vi "Autonomous Independent.vi"() -> ()   [LabVIEW 2015]
doc: "This VI is called when autonomous begins, and will automatically be terminated when autonomous ends. You can carry out timed or sensor driven robot movement independently without needing to return to the caller."
uses:
  Goal Selection.ctl
  Defense Position.ctl
  Defenses.ctl
  Auto 2 Control.ctl
  <vilib>/Platform/TimedLoop/XDataNode/timing_clust.ctl
  <vilib>/Platform/TimedLoop/XDataNode/nitl_modes.ctl
  <vilib>/Platform/TimedLoop/XDataNode/wakeup.ctl
  <vilib>/Rock Robotics/WPI/MotorControl/WPI_MotorControlDeviceRef.ctl
  <vilib>/Rock Robotics/WPI/MotorControl/WPI_MotorControlType.ctl
  <vilib>/Rock Robotics/SystemInterfaces/DIO/FPGA_DIOPWMChannel.ctl
  <vilib>/Rock Robotics/WPI/PWM/WPI_PWMDeadband.ctl
  <vilib>/Rock Robotics/WPI/CAN/Jaguar/SubVIs/WPI_CANJaguar_ControlMode.ctl
  <vilib>/Rock Robotics/WPI/CAN/TalonSRX/WPI_CANTalonSRX_APIControlMode.ctl
  <userlib>/836-Library/Drive/Drive Code/Drive Code Support/Drive Code Bundle.ctl
  <userlib>/836-Library/Drive/Drive Code/Drive Code Support/Sensor Cluster.ctl
  <userlib>/836-Library/Drive/Drive Code/Drive Code Support/Camera Cluster.ctl
  <userlib>/836-Library/Drive/Drive Code/Drive Code Support/Drive Code Notifier.ctl
  <userlib>/836-Library/Drive/Drive Code/Drive Code Support/Drive Code Command.ctl
  <userlib>/836-Library/Drive/Drive Code/Logging Data.ctl
  <userlib>/836-Library/Pneumatics/Support Code/Pneumatics Notifier.ctl
  <userlib>/836-Library/Pneumatics/Support Code/Pneumatics Command.ctl
  <userlib>/836-Library/Pneumatics/Support Code/Pneumatics Status.ctl
  PortcullisStates.ctl
  <userlib>/836-Library/System/TDMSv2/TDMS Channel Info.ctl
  <userlib>/836-Library/System/TDMSv2/TDMS RT FIFO Packet.ctl
  <vilib>/Rock Robotics/Network Tables/NT Read Number.vi
  <vilib>/Rock Robotics/Network Tables/NT Read Boolean.vi
  <userlib>/836-Library/Drive/Drive Code/Drive Code Support/Drive Loop Do Nothing.vi
  <userlib>/836-Library/Pneumatics/Support Code/Pneumatics Command Set Periodic.vi
  <userlib>/836-Library/Drive/Drive Code/Drive Code Support/Drive Loop Drive Distance.vi
  <userlib>/836-Library/Drive/Drive Code/Drive Code Support/Drive Loop Drive Continuous.vi
  <userlib>/836-Library/Drive/Drive Code/Drive Code Support/Drive Loop Turn.vi
  <userlib>/836-Library/Drive/Drive Code/Drive Code Support/Drive Loop Hold Yaw.vi
  <userlib>/836-Library/Drive/Drive Code/Drive Code Support/Drive Loop Follow Camera.vi
  <userlib>/836-Library/Drive/Drive Code/Drive Code Support/Drive Loop Hold Position.vi
  <vilib>/platform/TimedLoop/XDataNode/XDataNode.xnode
  <vilib>/Platform/TimedLoop/XDataNode/XDNodeRunTimeDep.lvlib
panel:
  out "Y":dbl
  out "Desired X pos":dbl
  out "X pos":dbl
  out "XY Current":cluster{"X":dbl, "Y":dbl}={"X"=133.11, "Y"=0.0}
  out "Pitch":dbl(graph)=0.125
  out "Initial Pitch":dbl=1.25
  out "Stable Over Pitch":bool
  out "Over Pitch Th":bool
  out "Over Encoder Distance":bool
  out "Camera Valid":bool
  out "Robot Pitch":dbl
  out "Current Angle":dbl=-0.5625
  out "Desired Angle":dbl
  out "Initial Encoder Distance":dbl
  out "Current Distance":dbl=136.322655
  out "Target Distance":dbl
  out "Waveform Chart":dbl(graph)=19.0
  in  "Return Point":cluster{"X":dbl, "Y":dbl}
  in  "Tab Control":enum32{"Auto 2"}(tab)
  in  "Score Intake timer":dbl=3.0
  out "Defense to Cross":T1=enum."Portcullis"
  out "Starting Position":T2=enum."3"
  out "Goal Target":T3=enum."Stop"
  out "Starting IMU Yaw":dbl
  out "Current State":T4=enum."Stop"
  out "Pitch Up Detected":bool
  out "Pitch Down Detected":bool
  in  "Override Pitch Detection":bool
  in  "Backup Power":dbl=-1.0 format="%#_13g"
  in  "Tower Backup Offset":dbl=48.0 format="%#_13g"
  in  "Dist from Def":dbl=60.0
  in  "Portcullis Point":dbl=100.0
  in  "Portcullis Cross Power":dbl=0.6
  in  "Encoder Pause":dbl=0.4
  in  "Dist cross":dbl=120.0
  in  "Encoder not moving val":dbl=0.001
  in  "Eval Period for Port":dbl=0.8 format="%#_13g"
  # "00 - Start Delay\n01 - Defense Selection\n02 - Defense Crossing Detection\n03 - Drive Forward Past Defense\n04 - Turn to Rally Pt\n05 - Complete Rally pt Turn\n06 - Drive to Rally Pt\n07 - Finish Rally Pt Turn\n08 - Turn to Tower\n09 - Complete Turn to Tower\n10 - Drive to Twoer\n11 - Compelte Drive to Tower\n12 - Score\n13 - Back to Defense\n14 - Stop"
  # "Starting Values"
  # "Values from Dash"
  # "To Dash"
  # "TO QCP"
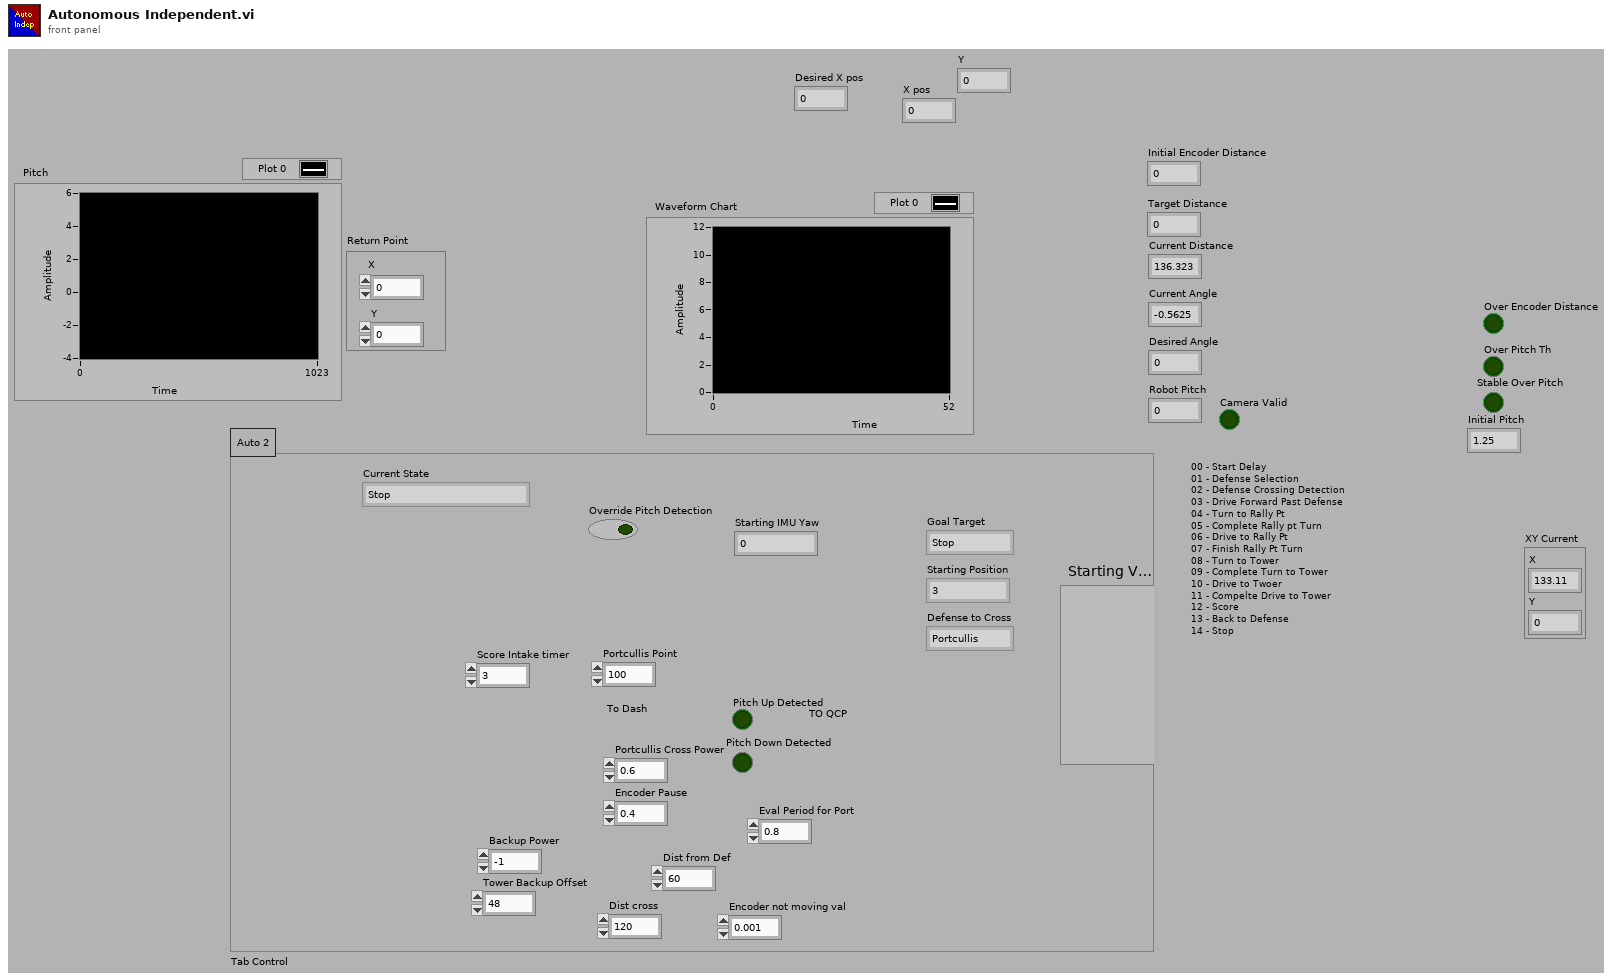
[diagram p1: front panel]
types:
  T1 = typedef "Defenses.ctl" = enum16{"Low Bar", "Rough Terrain", "Moat", "Rock Wall", "Cheval de Frise", "Portcullis", "Sally Port", "Drawbridge", "Ramparts"}
  T2 = typedef "Defense Position.ctl" = enum16{"1", "2", "3", "4", "5"}
  T3 = typedef "Goal Selection.ctl" = enum16{"Left Goal", "Right Goal", "Stop"}
  T4 = typedef "Auto 2 Control.ctl" = enum16{"Start Delay", "Defense Selection", "Defense Crossing Detection", "Drive Forward Past Defense", "Turn to Rally Pt", "Complete Rally Pt Turn", "Drive to Rally Pt", "Finish Drive to Rally Pt", "Turn to Tower", "Complete Turn to Tower", "Drive to Tower", "Complete Drive to Tower", "Score", "Parallel to Position", "Finish Backing Parallel to Pos", "Turn to Defense ", "Finish Turn to Def", "Back to Defense", "Finish Back to Defense", "Stop"}
  T5 = typedef "TDMS Channel Info.ctl" = cluster{"TDMS Data":T6, "TDMS RT FIFO":refnum<k33>}
  T6 = typedef "TDMS RT FIFO Packet.ctl" = cluster{"Group/CMD":i32, "Channel":i32, "Data":dbl}
  T7 = typedef "PortcullisStates.ctl" = enum16{"Drive up to Portcullis", "Intake Up", "Pause", "Cross", "Finish Cross"}
  T8 = typedef "WPI_MotorControlDeviceRef.ctl" = cluster{"DeviceStatus":errorcluster, "Type":T9, "PWM":cluster{"PWM Channel":T10, "DeadBand":T11}, "CAN":cluster{"Device Number":u8, "Control Mode":T12, "Semaphore":T13, "Max Vout":dbl, "TalonSRX Control Mode":T14}, "Invert":bool}
  T9 = typedef "WPI_MotorControlType.ctl" = enum16{"PWM", "CAN", "CANTalonSRX"}
  T10 = typedef "FPGA_DIOPWMChannel.ctl" = enum8{"PWM 0", "PWM 1", "PWM 2", "PWM 3", "PWM 4", "PWM 5", "PWM 6", "PWM 7", "PWM 8", "PWM 9", "PWM MXP 0", "PWM MXP 1", "PWM MXP 2", "PWM MXP 3", "PWM MXP 4", "PWM MXP 5", "PWM MXP 6", "PWM MXP 7", "PWM MXP 8", "PWM MXP 9", "Invalid"}
  T11 = typedef "WPI_PWMDeadband.ctl" = cluster{"Name":string, "maxPositivePwm":i32, "minPositivePwm":i32, "centerPwm":i32, "maxNegativePwm":i32, "minNegativePwm":i32, "angularRange":u16}
  T12 = typedef "WPI_CANJaguar_ControlMode.ctl" = enum8{"Percent VBus", "Current", "Speed", "Position", "Voltage"}
  T13 = typedef "Semaphore RefNum" = refnum<k1>
  T14 = typedef "WPI_CANTalonSRX_APIControlMode.ctl" = enum8{"Percent VBus", "Speed", "Position", "Slave", "Unchanged / Invalid", "Voltage Compensation", "Current", "Motion Profile"}
  T15 = typedef "Drive Code Bundle.ctl" = cluster{"Sensor Data":T16, "Drive Command rt fifo":refnum<k33>, "Logging Data":refnum<k33>}
  T16 = typedef "Sensor Cluster.ctl" = cluster{"Gyro Data":cluster{"Gyro RT FIFO":refnum<k33>, "Gyro Current":dbl, "Gyro Hold":dbl}, "Encoder Data":cluster{"Encoder RT FIFO":refnum<k33>, "Encoder Current":dbl, "Encoder Hold":dbl}, "Camera Data":cluster{"Camera RT FIFO":refnum<k33>, "Camera Current":T17}}
  T17 = typedef "Camera Cluster.ctl" = cluster{" Angle":dbl, "Valid":bool}
  T18 = typedef "Pneumatics Notifier.ctl" = cluster{"Command":refnum<notifier>, "Status":refnum<queue>}
  T19 = cluster{"intakeMotor":T8, "IMU Pitch":dbl, "Goal Target":T3, "IMU Yaw":dbl, "Initial Time":dbl, "Defense To Cross":T1, "Initial Position":T2, "Return Point":cluster{"X":dbl, "Y":dbl}, "Leave Tower?":bool, "Starting Delay":dbl, "IMU Roll":dbl, "Return Position":T2, "Drive Loop Cluster":T15, "Intake Command Cluster":T18}
  T20 = typedef "XDNodeRunTimeDep.lvlib/timing_clust.ctl" = cluster{"Expected End [f-1]":u64, "Actual End [f-1]":u64, "Finished Late? [f-1]":bool, "Expected End [i-1]":u64, "Actual End [i-1]":u64, "Finished Late? [i-1]":bool, "Expected Start [i]":u64, "Actual Start [i]":u64, "Expected Start [f]":u64, "Actual Start [f]":u64, "Source Name":string, "Structure Name":string, "Period":i64, "Deadline":i64, "Offset":i64, "Start":i64, "Priority":i32, "Timeout":i32, "Mode":T21, "Wakeup Reason":T22, "Error":errorcluster, "Source Type":string, "Secondary Source Type":string, "Global End Time":u64, "Global Start Time":u64, "Frame Duration":u64, "Iteration Duration":u64, "Assigned CPU":i32, "I/O Scan Engine Mode":u32}
  T21 = typedef "XDNodeRunTimeDep.lvlib/nitl_modes.ctl" = enum32{"No Change", "Process missed periods, maintain original phase", "Discard missed periods, maintain original phase", "Process missed periods, ignore original phase", "Discard missed periods, ignore original phase"}
  T22 = typedef "XDNodeRunTimeDep.lvlib/wakeup.ctl" = enum32{"Normal", "Aborted", "Asynchronous wakeup", "Timing source error", "Timed loop error", "Timeout"}
  T23 = typedef "Pneumatics Command.ctl" = enum16{"Nothing", "Forward", "Reverse", "Toggle"}
  T24 = cluster{"Rally Pt 2 X L":dbl, "Rally Pt 2 X L":dbl}
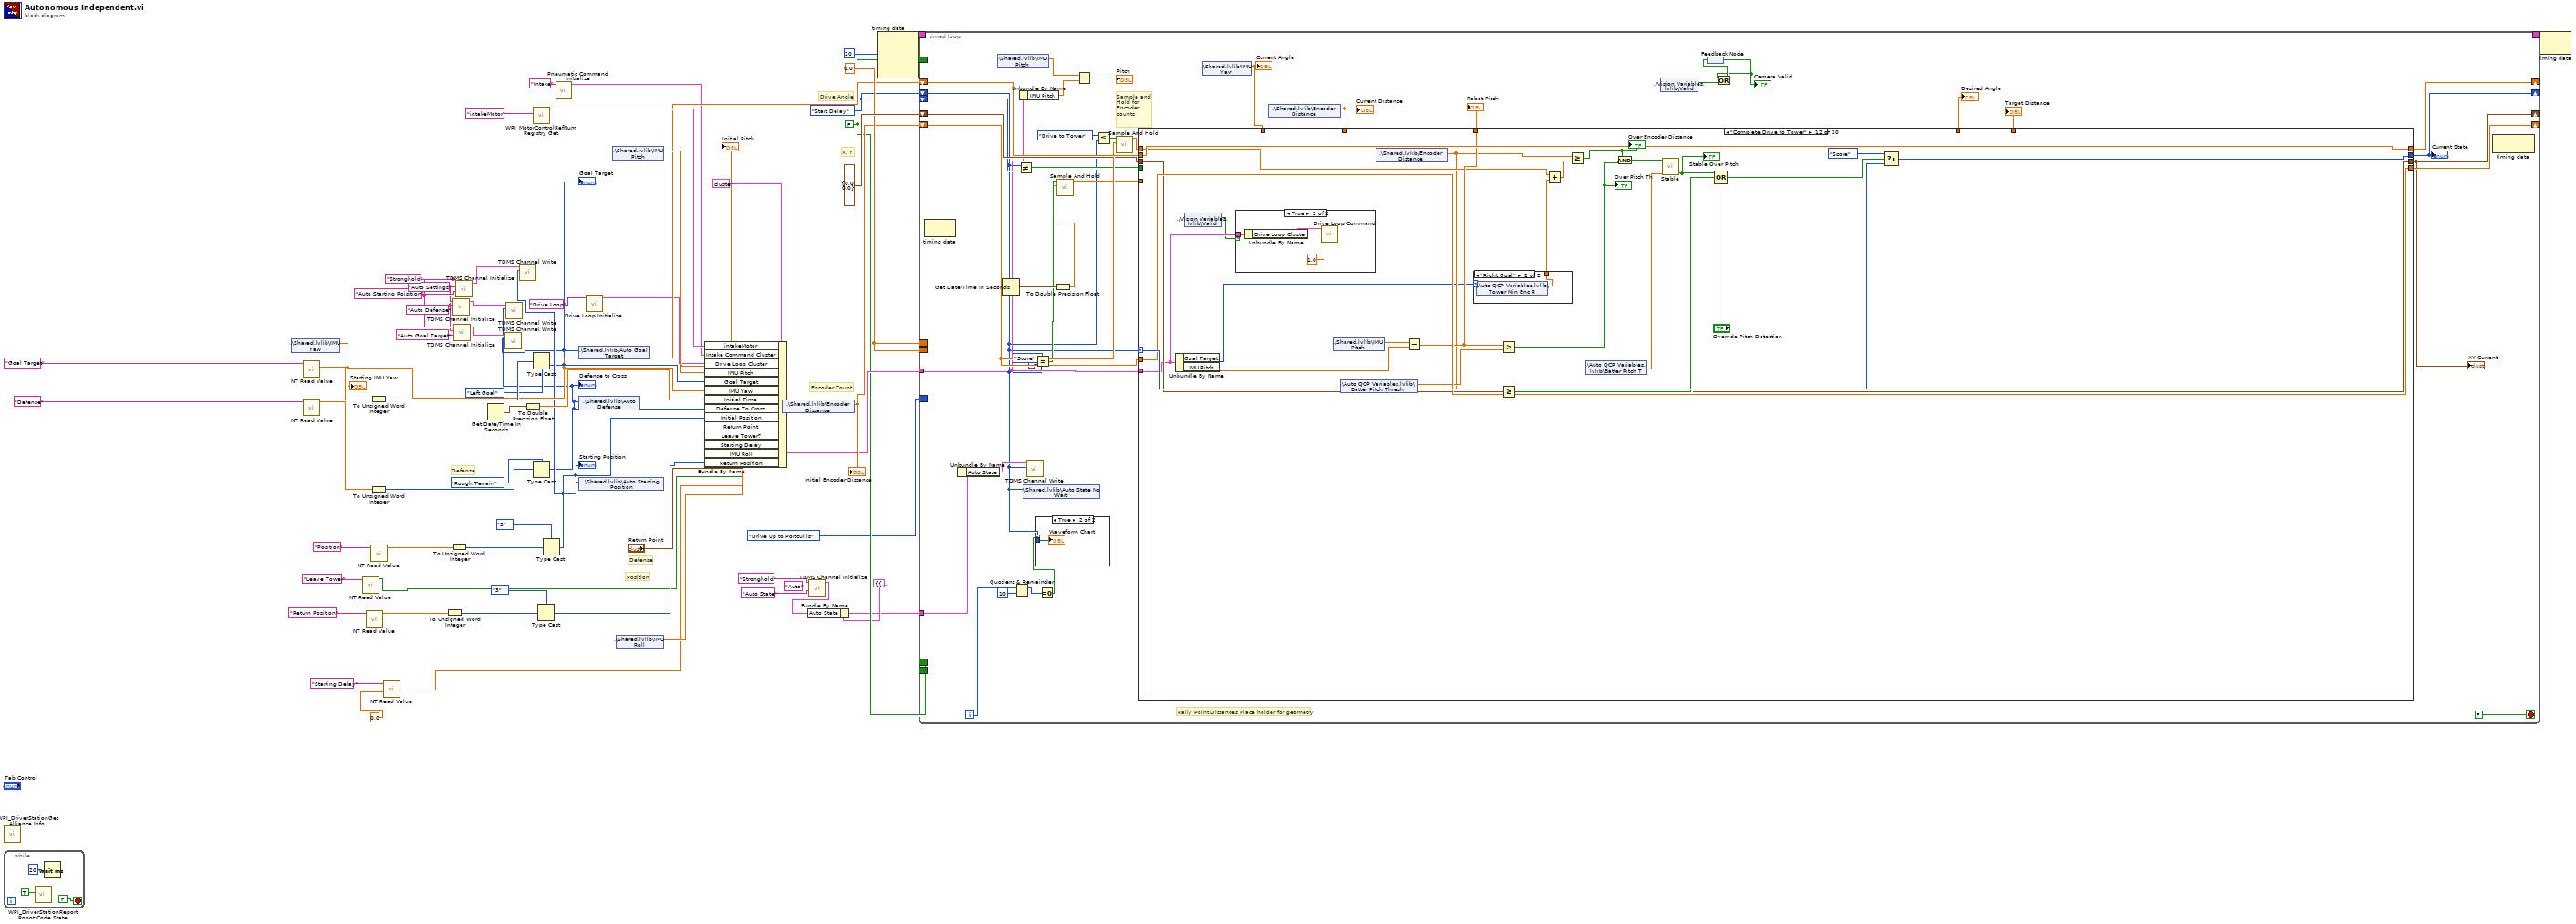
[diagram p0: block diagram]
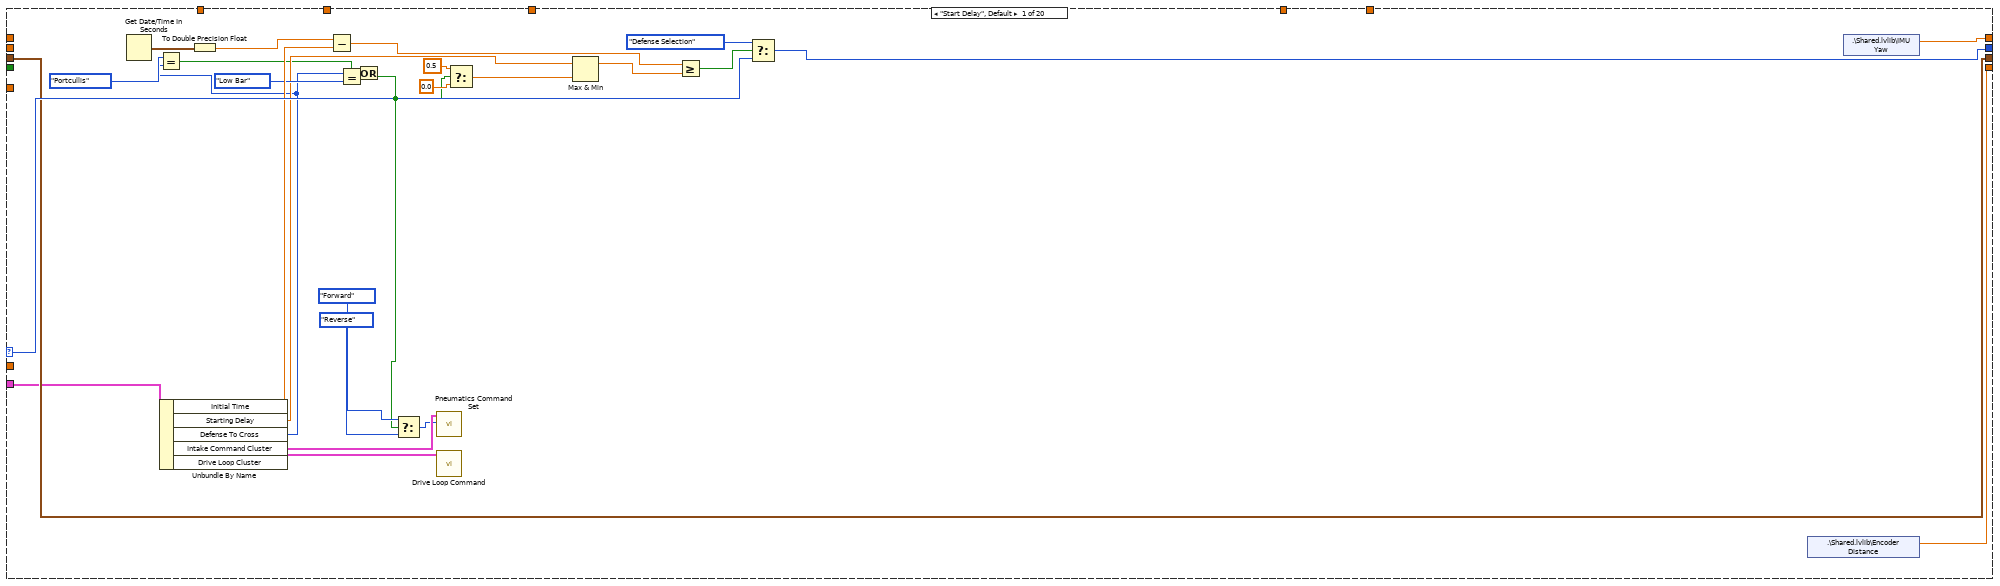
[diagram p3: hidden frame]
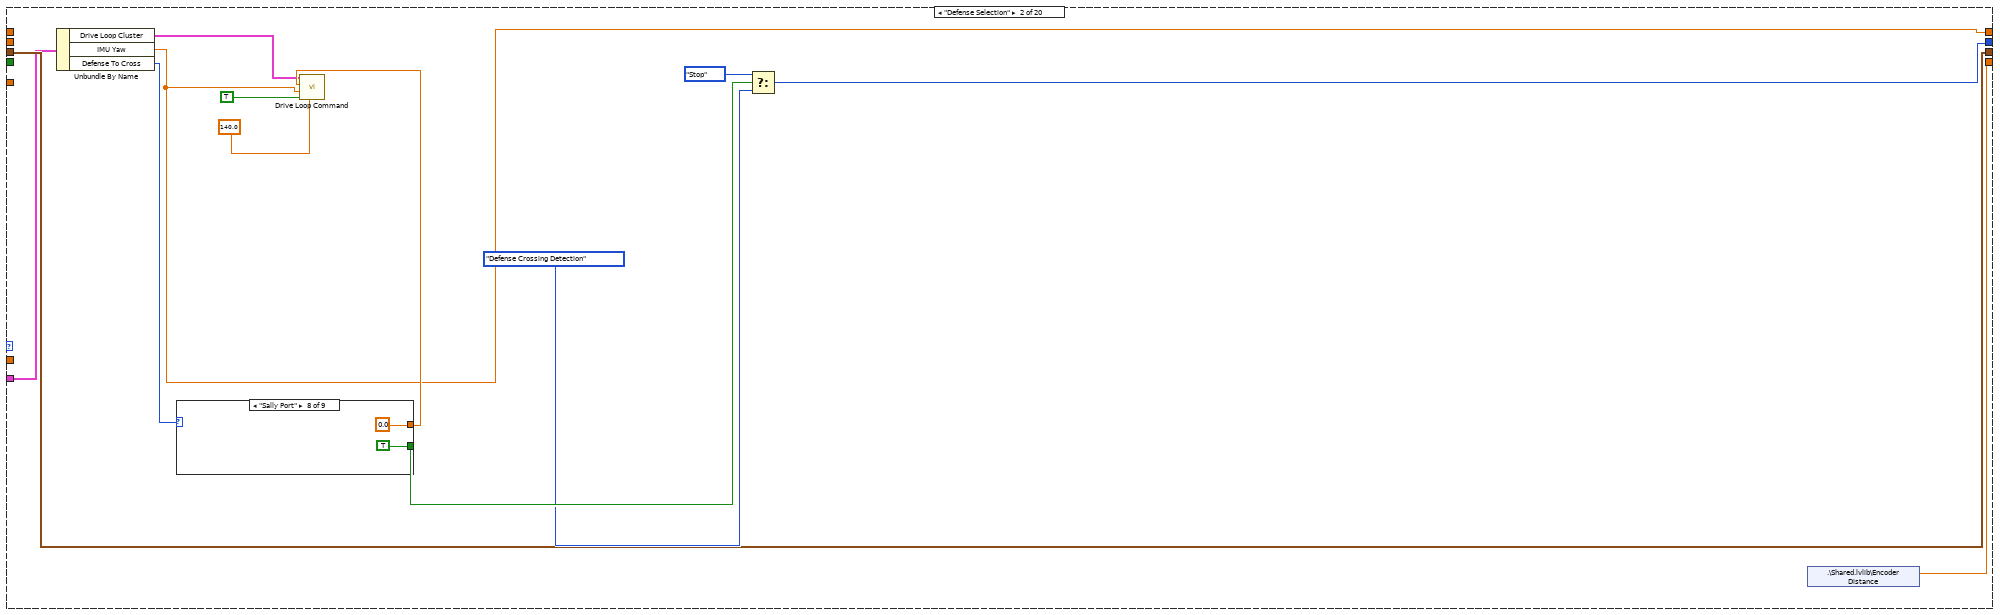
[diagram p4: hidden frame]
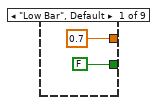
[diagram p5: hidden frame]
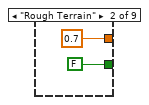
[diagram p6: hidden frame]
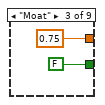
[diagram p7: hidden frame]
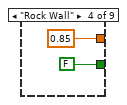
[diagram p8: hidden frame]
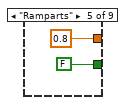
[diagram p9: hidden frame]
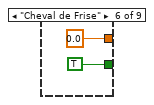
[diagram p10: hidden frame]
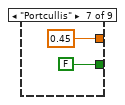
[diagram p11: hidden frame]
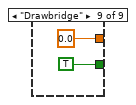
[diagram p12: hidden frame]
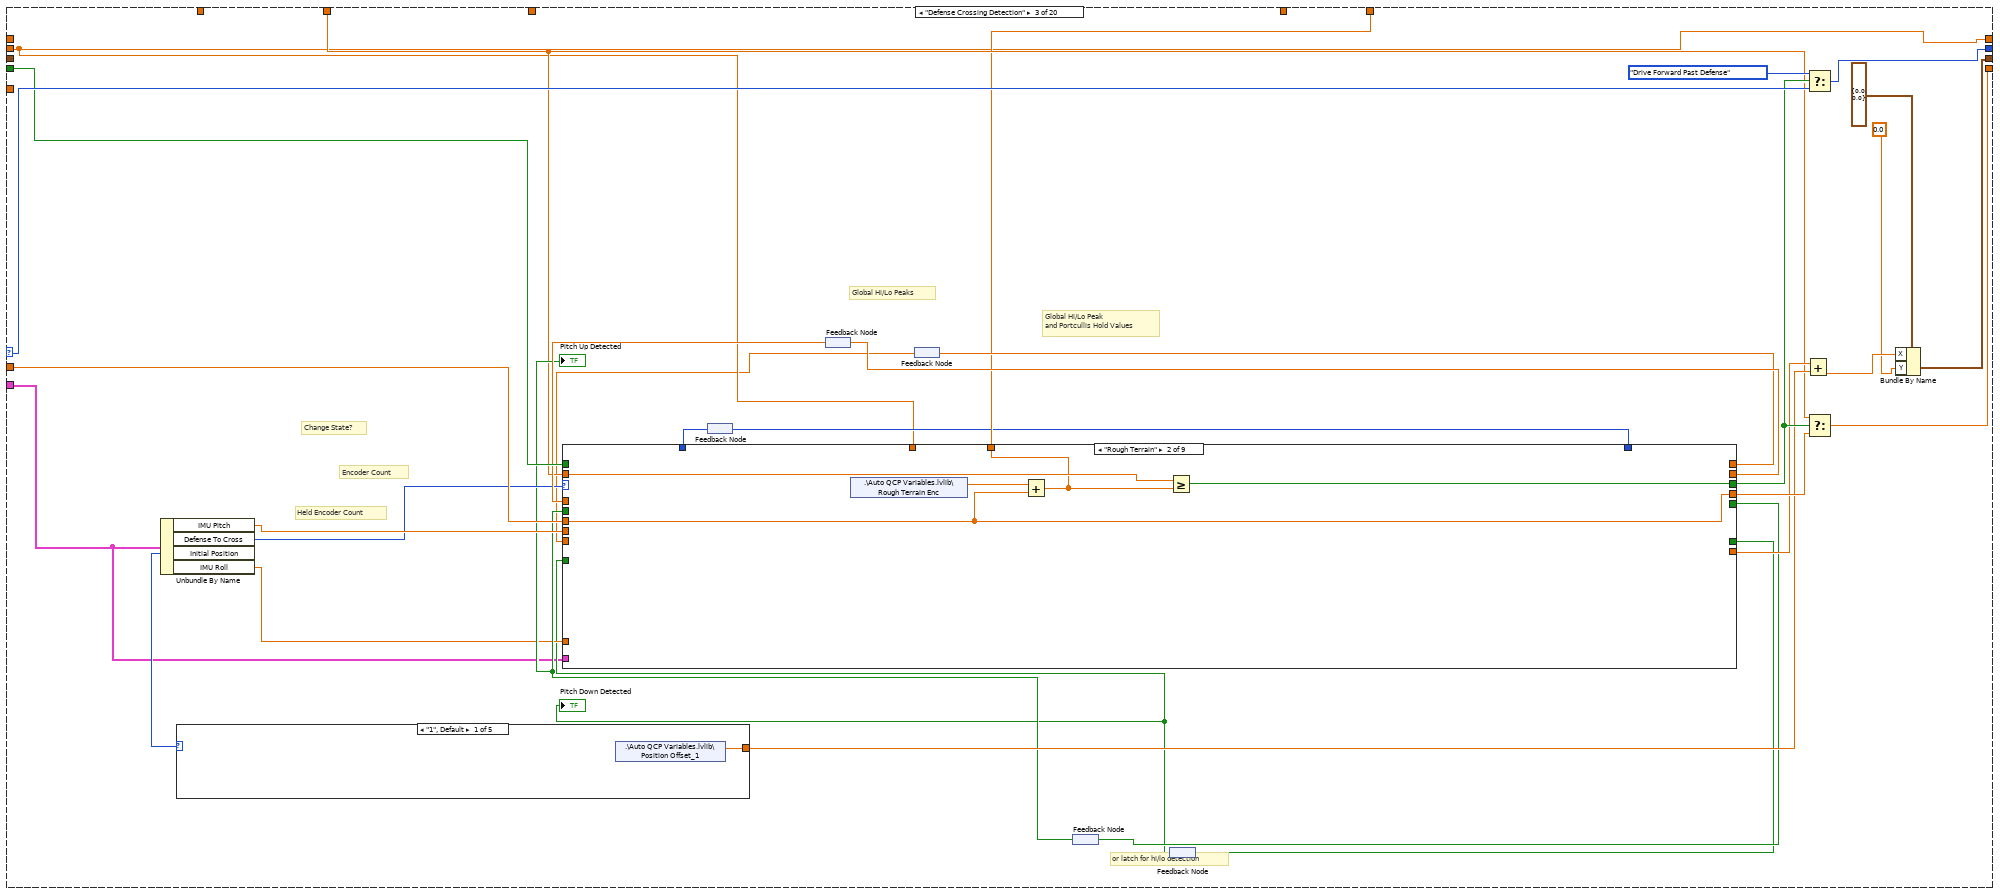
[diagram p13: hidden frame]
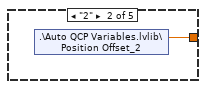
[diagram p14: hidden frame]
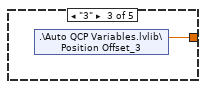
[diagram p15: hidden frame]
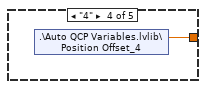
[diagram p16: hidden frame]
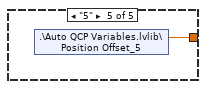
[diagram p17: hidden frame]
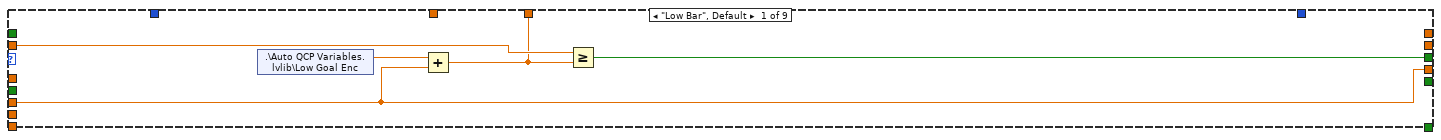
[diagram p18: hidden frame]
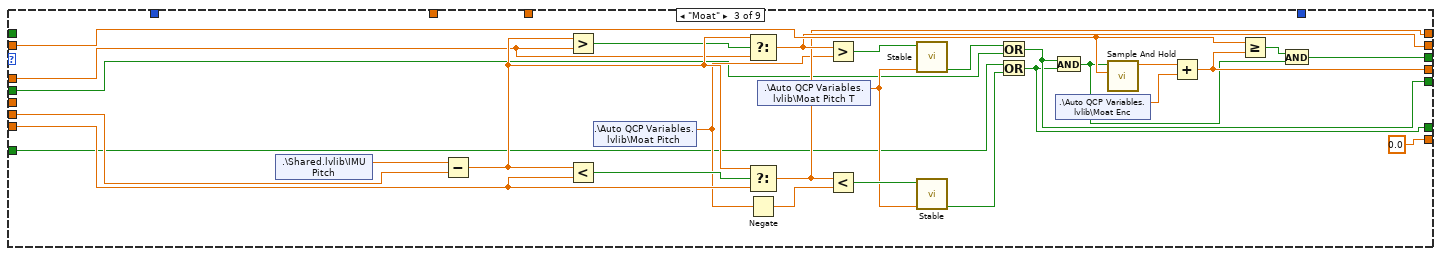
[diagram p19: hidden frame]
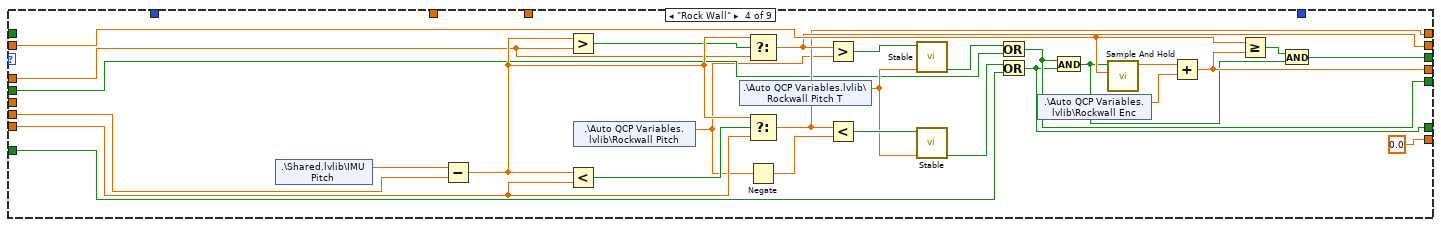
[diagram p20: hidden frame]
diagram:
  w9 = "Auto Settings" ("Group")
  w10 = "Stronghold" ("TDMS Name")
  w33 = FALSE
  w44 = 0.0 ("Double")
  w43 = Auto_2_Control."Start Delay"
  # "X, Y"
  # "Drive Angle"
  # "Encoder Count"
  # "Position"
  # "Defense"
  # "Defense"
  n1 = call <vilib>:"WPI_DriverStationGet Alliance Info.vi"() -> ()  [unwired: 12 out]
  n2 = while {
    stop <- FALSE stop-if-true
    n3 = call <vilib>:"WPI_DriverStationReport Robot Code State.vi"("Autonomous"=TRUE) -> ()  [unwired: 10 in, 1 out]
    n4 = Wait (ms)(milliseconds to wait=u32 20) -> ()  [unwired: 1 out]
  }
  n5 = shared-variable ".\\Shared.lvlib\\IMU Yaw"() -> (w37:dbl)  [unwired: 1 in, 1 out]
  "Starting IMU Yaw" <- w37
  n6 = call-poly <vilib>:"NT Read Value.vi"("Name"="Goal Target") -> ("Numeric"=w54:dbl)  [unwired: 9 in, 1 out]
  n7 = call-poly <vilib>:"NT Read Value.vi"("Name"="Defense") -> ("Numeric"=w60:dbl)  [unwired: 9 in, 1 out]
  n8 = call-poly <vilib>:"NT Read Value.vi"("Name"="Leave Tower") -> ("Boolean"=w27:bool)  [unwired: 9 in, 1 out]
  n9 = call-poly <vilib>:"NT Read Value.vi"("Name"="Return Position") -> ("Numeric"=w29:dbl)  [unwired: 9 in, 1 out]
  n10 = To Unsigned Word Integer(number=w54) -> (unsigned 16bit integer=w55:u16)
  n11 = To Unsigned Word Integer(number=w60) -> (unsigned 16bit integer=w59:u16)
  n12 = call-poly <vilib>:"NT Read Value.vi"("Name"="Position") -> ("Numeric"=w52:dbl)  [unwired: 9 in, 1 out]
  n13 = call-poly <vilib>:"NT Read Value.vi"("Default Value"=0.0, "Name"="Starting Delay") -> ("Numeric"=w23:dbl)  [unwired: 8 in, 1 out]
  n14 = To Unsigned Word Integer(number=w29) -> (unsigned 16bit integer=w31:u16)
  n15 = To Unsigned Word Integer(number=w52) -> (unsigned 16bit integer=w50:u16)
  n16 = call <userlib>:"TDMS Channel Initialize.vi"("Channel"="Auto Defense", "Group"=w9, "TDMS"=w10) -> ("TDMS Channel Info"=w5:T5)  [unwired: 8 in]
  n17 = call <userlib>:"TDMS Channel Initialize.vi"("Channel"="Auto Goal Target", "Group"=w9, "TDMS"=w10) -> ("TDMS Channel Info"=w4:T5)  [unwired: 8 in]
  n18 = call <userlib>:"TDMS Channel Initialize.vi"("Channel"="Auto Starting Poisition", "Group"=w9, "TDMS"=w10) -> ("TDMS Channel Info"=w6:T5)  [unwired: 8 in]
  n19 = Get Date/Time In Seconds() -> (seconds since 1Jan1904=w48:timestamp)
  n20 = To Double Precision Float(number=w48) -> (double precision float=w36:dbl)
  n21 = call <vilib>:"WPI_MotorControlRefNum Registry Get.vi"("refnum name"="intakeMotor") -> ("MotorControlDevRef"=w40:T8)  [unwired: 9 in, 1 out]
  n22 = Type Cast(type=Goal_Selection."Left Goal" ("Goal Target"), x=w55) -> (*(type *) &x=w1:T3)
  "Goal Target" <- w1
  n23 = call <userlib>:"TDMS Channel Write.vi"("Data"=w1, "TDMS Channel Info in"=w4) -> ()  [unwired: 9 in, 1 out]
  n24 = Type Cast(type=Defenses."Rough Terrain", x=w59) -> (*(type *) &x=w2:T1)
  "Defense to Cross" <- w2
  n25 = call <userlib>:"TDMS Channel Write.vi"("Data"=w2, "TDMS Channel Info in"=w5) -> ()  [unwired: 9 in, 1 out]
  n26 = Type Cast(type=Defense_Position."3", x=w31) -> (*(type *) &x=w28:T2)
  n27 = Type Cast(type=Defense_Position."3", x=w50) -> (*(type *) &x=w3:T2)
  "Starting Position" <- w3
  n28 = call <userlib>:"TDMS Channel Write.vi"("Data"=w3, "TDMS Channel Info in"=w6) -> ()  [unwired: 9 in, 1 out]
  n29 = call <userlib>:"Pneumatic Command Initialize.vi"("name (unnamed)"="Intake") -> ("Pneumatic Command Cluster"=w18:T18)  [unwired: 9 in, 1 out]
  n30 = shared-variable ".\\Shared.lvlib\\Auto Goal Target"(w1) -> ()  [unwired: 1 in, 1 out]
  n31 = shared-variable ".\\Shared.lvlib\\Auto Defense"(w2) -> ()  [unwired: 1 in, 1 out]
  n32 = shared-variable ".\\Shared.lvlib\\Auto Starting Position"(w3) -> ()  [unwired: 1 in, 1 out]
  n33 = call <userlib>:"Drive Loop Initialize.vi"("name (unnamed)"="Drive Loop") -> ("Drive Loop Cluster"=w21:T15)  [unwired: 9 in, 1 out]
  n34 = shared-variable ".\\Shared.lvlib\\IMU Pitch"() -> (w38:dbl)  [unwired: 1 in, 1 out]
  "Initial Pitch" <- w38
  n35 = shared-variable ".\\Shared.lvlib\\IMU Roll"() -> (w34:dbl)  [unwired: 1 in, 1 out]
  n36 = Bundle By Name(cluster=T19 {"intakeMotor"={"DeviceStatus"={"status"=FALSE, "code"=0, "source"=""}, "Type"=enum."PWM", "PWM"={"PWM Channel"=enum."Invalid", "DeadBand"={"Name"="", "maxPositivePwm"=0, "minPositivePwm"=0, "centerPwm"=0, "maxNegativePwm"=0, "minNegativePwm"=0, "angularRange"=0}}, "CAN"={"Device Number"=0, "Control Mode"=enum."Percent VBus", "Semaphore"=refnum, "Max Vout"=12.0, "TalonSRX Control Mode"=enum."Percent VBus"}, "Invert"=FALSE}, "IMU Pitch"=0.0, "Goal Target"=enum."Left Goal", "IMU Yaw"=0.0, "Initial Time"=0.0, "Defense To Cross"=enum."Low Bar", "Initial Position"=enum."3", "Return Point"={"X"=0.0, "Y"=0.0}, "Leave Tower?"=FALSE, "Starting Delay"=0.0, "IMU Roll"=0.0, "Return Position"=enum."3", "Drive Loop Cluster"={"Sensor Data"={"Gyro Data"={"Gyro RT FIFO"=refnum, "Gyro Current"=0.0, "Gyro Hold"=0.0}, "Encoder Data"={"Encoder RT FIFO"=refnum, "Encoder Current"=0.0, "Encoder Hold"=0.0}, "Camera Data"={"Camera RT FIFO"=refnum, "Camera Current"={" Angle"=0.0, "Valid"=FALSE}}}, "Drive Command rt fifo"=refnum, "Logging Data"=refnum}, "Intake Command Cluster"={"Command"=refnum, "Status"=refnum}}, "intakeMotor"=w40, "Intake Command Cluster"=w18, "Drive Loop Cluster"=w21, "IMU Pitch"=w38, "Goal Target"=w1, "IMU Yaw"=w37, "Initial Time"=w36, "Defense To Cross"=w2, "Initial Position"=w3, "Return Point"="Return Point", "Leave Tower?"=w27, "Starting Delay"=w23, "IMU Roll"=w34, "Return Position"=w28) -> (w39:T19)
  n37 = shared-variable ".\\Shared.lvlib\\Encoder Distance"() -> (w42:dbl)  [unwired: 1 in, 1 out]
  "Initial Encoder Distance" <- w42
  n38 = call <userlib>:"TDMS Channel Initialize.vi"("Channel"="Auto State", "Group"="Auto", "TDMS"="Stronghold" ("TDMS Name")) -> ("TDMS Channel Info"=w15:T5)  [unwired: 8 in]
  n39 = Bundle By Name(cluster=cluster{"Auto State":T5} {"Auto State"={"TDMS Data"={"Group/CMD"=0, "Channel"=0, "Data"=0.0}, "TDMS RT FIFO"=refnum}}, "Auto State"=w15) -> (w14:cluster{"Auto State":T5})
  n40 = node-c288(i64 20 ("Period")) -> (w47:T20)  [unwired: 3 in]
  n41 = timed-loop {
    timing: w47 -> [_]
    timing-out: [_] -> w46
    shift-right: [w92] -> _
    shift-left: w43 -> [w66]
    shift-right: [w102] -> _
    shift-left: w42 -> [w99]
    shift-right: [w100] -> _
    shift-left: w37 -> [w101]
    shift-right: [w95] -> _
    shift-left: cluster{"X":dbl, "Y":dbl} {"X"=0.0, "Y"=0.0} ("input cluster") -> [w96]
    shift-left: w43 -> [w94]
    border: w44 -> [_]
    border: w44 -> [_]
    tunnel: w39 -> [w78]
    border: w33 -> [_]
    border: w33 -> [_]
    border: w33 -> [_]
    border: PortcullisStates."Drive up to Portcullis" -> [_]
    tunnel: w14 -> [w68]
    i -> [w86]
    stop <- FALSE stop-if-true
    # "Sample and Hold for Encoder counts"
    # "Rally Point Distances Place holder for geometry"
    n42 = node-c288() -> ()  [unwired: 1 in, 1 out]
    n43 = Unbundle By Name(w68) -> ("Auto State"=w67:T5)
    n44 = shared-variable ".\\Shared.lvlib\\IMU Pitch"() -> (w77:dbl)  [unwired: 1 in, 1 out]
    n45 = Get Date/Time In Seconds() -> (seconds since 1Jan1904=w72:timestamp)
    n46 = Quotient & Remainder(x=w86, y=10) -> (x-y*floor(x/y)=w84:i32)  [unwired: 1 out]
    n47 = Not Equal?(x=w66, y=w94) -> (x != y?=w73:bool)
    n48 = Unbundle By Name(w78) -> ("IMU Pitch"=w76:dbl)
    n49 = shared-variable ".\\Shared.lvlib\\Auto State No Wait"(w66) -> ()  [unwired: 1 in, 1 out]
    n50 = call <userlib>:"TDMS Channel Write.vi"("Data"=w66, "TDMS Channel Info in"=w67) -> ()  [unwired: 9 in, 1 out]
    n51 = Equal?(x=w66, y=Auto_2_Control."Score") -> (x = y?=w69:bool)
    n52 = Equal To 0?(x=w84) -> (x = 0?=w83:bool)
    n53 = case shown="True" w83 {
      tunnel: w66 -> [_ w103]
      frame False {
      }
      frame True {
        "Waveform Chart" <- w103
      }
    }
    n54 = To Double Precision Float(number=w72) -> (double precision float=w71:dbl)
    n55 = call "Sample And Hold.vi"("Signal"=w71, "Condition"=w69) -> ("Signal Out"=w70:dbl)  [unwired: 9 in]
    n56 = Subtract(x=w77, y=w76) -> (x-y=→"Pitch":dbl)
    n57 = Less Or Equal?(x=Auto_2_Control."Drive to Tower", y=w66) -> (x <= y?=w93:bool)
    n58 = call "Sample And Hold.vi"("Signal"=w99, "Condition"=w93) -> ("Signal Out"=w98:dbl)  [unwired: 9 in]
    n59 = shared-variable ".\\Shared.lvlib\\IMU Yaw"() -> (w74:dbl)  [unwired: 1 in, 1 out]
    "Current Angle" <- w74
    n60 = shared-variable ".\\Shared.lvlib\\Encoder Distance"() -> (w89:dbl)  [unwired: 1 in, 1 out]
    "Current Distance" <- w89
    n61 = case shown="\"Complete Drive to Tower\"" w66 {
      selector: w66 -> [w127 _ w194 w377 _ w479 _ w502 _ w535 _ w574 w600 _ w627 _ w670 _ w703 _]
      tunnel: [w126 w141 w193 w376 w434 w482 Auto_2_Control."Finish Drive to Rally Pt" ("t") w504 Auto_2_Control."Complete Turn to Tower" ("t") w534 Auto_2_Control."Complete Drive to Tower" ("t") w573 w599 Auto_2_Control."Finish Backing Parallel to Pos" w634 Auto_2_Control."Finish Turn to Def" w672 Auto_2_Control."Finish Back to Defense" ("t") w701 Auto_2_Control."Stop"] -> w92
      tunnel: [w123 w140 w188 w372 w433 w478 w491 w498 w521 w533 w548 w566 w591 w613 w630 w658 w668 w690 w699 w711] -> w102
      tunnel: w99 -> [_ _ w191 w372 _ _ w495 w498 _ _ _ w566 _ w613 w630 _ _ w692 w699 w711]
      tunnel: [w122 w132 w165 w362 w418 w474 w488 w500 w508 w536 w547 w564 w592 w608 w622 w656 w669 w688 w700 w712] -> w100
      tunnel: w101 -> [_ _ w165 _ _ w474 w488 w500 _ w536 w547 w564 _ w608 w622 _ w669 w688 w700 w712]
      tunnel: w98 -> [_ _ _ _ _ _ _ _ _ _ _ w557 _ _ _ _ _ _ _ _]
      tunnel: w96 -> [w124 w139 _ w363 w432 w477 w494 w497 w510 w530 w546 w560 w590 w612 w632 w667 w683 w693 w704 w713]
      tunnel: [w124 w139 w186 w370 w421 w477 w494 w497 w509 w530 w546 w560 w590 w612 w631 w667 w683 w694 w704 w713] -> w95
      tunnel: w73 -> [_ _ w181 _ _ _ _ _ _ _ _ _ w581 _ _ _ _ _ _ w707]
      tunnel: w78 -> [w121 w138 w163 w367 w431 _ w492 _ w519 _ w544 w552 w586 w614 w640 w666 w681 w695 _ w709]
      tunnel: w89 -> [_ _ w169 _ _ _ _ _ _ _ _ _ _ _ w644 w658 _ _ w698 _]
      tunnel: [_ _ w168 w364 _ _ w491 _ _ _ _ _ _ _ _ _ _ _ w699 _] -> w88
      tunnel: [_ _ _ w362 w418 w474 _ _ _ _ _ _ _ _ _ _ _ _ _ _] -> w87
      tunnel: [_ _ _ _ _ _ _ _ _ _ _ w559 _ _ _ _ _ _ _ _] -> w82
      tunnel: w74 -> [_ _ _ _ _ _ _ _ _ _ _ _ _ _ _ _ w682 _ _ _]
      tunnel: w70 -> [_ _ _ _ _ _ _ _ _ _ _ _ w582 _ _ _ _ _ _ _]
      frame "Start Delay", Default {
        n62 = Get Date/Time In Seconds() -> (seconds since 1Jan1904=w131:timestamp)
        n63 = Unbundle By Name(w121) -> ("Initial Time"=w120:dbl, "Starting Delay"=w115:dbl, "Defense To Cross"=w111:T1, "Intake Command Cluster"=w108:T18, "Drive Loop Cluster"=w109:T15)
        n64 = Equal?(x=Defenses."Portcullis" ("y"), y=w111) -> (x = y?=w110:bool)
        n65 = To Double Precision Float(number=w131) -> (double precision float=w130:dbl)
        n66 = Subtract(x=w130, y=w120) -> (x-y=w129:dbl)
        n67 = Equal?(x=w111, y=Defenses."Low Bar") -> (x = y?=w113:bool)
        n68 = Or(x=w110, y=w113) -> (x .or. y?=w104:bool)
        n69 = Select(t=Pneumatics_Command."Forward" ("Solenoid Command"), s=w104, f=Pneumatics_Command."Reverse" ("Solenoid Command")) -> (s? t:f=w107:T23)
        n70 = call-poly <userlib>:"Pneumatics Command Set.vi"("Solenoid Command"=w107, "Cluster"=w108) -> ()  [unwired: 9 in, 1 out]
        n71 = call-poly <userlib>:"Drive Loop Command.vi"("Drive Loop Cluster"=w109) -> ()  [unwired: 11 in]
        n72 = Select(t=0.5, s=w104, f=0.0) -> (s? t:f=w116:dbl)
        n73 = Max & Min(x=w115, y=w116) -> (max(x,y)=w114:dbl)  [unwired: 1 out]
        n74 = Greater Or Equal?(x=w129, y=w114) -> (x >= y?=w128:bool)
        n75 = Select(t=Auto_2_Control."Defense Selection", s=w128, f=w127) -> (s? t:f=w126:T4)
        n76 = shared-variable ".\\Shared.lvlib\\Encoder Distance"() -> (w123:dbl)  [unwired: 1 in, 1 out]
        n77 = shared-variable ".\\Shared.lvlib\\IMU Yaw"() -> (w122:dbl)  [unwired: 1 in, 1 out]
      }
      frame "Defense Selection" {
        n78 = Unbundle By Name(w138) -> ("Drive Loop Cluster"=w134:T15, "IMU Yaw"=w132:dbl, "Defense To Cross"=w137:T1)
        n79 = case shown="\"Sally Port\"" w137 {
          tunnel: [0.7 ("Power") 0.7 ("Power") 0.75 ("Power") 0.85 ("Power") 0.8 ("Power") 0.0 ("Power") 0.45 ("Power") 0.0 ("Power") 0.0 ("Power")] -> w135
          tunnel: [FALSE FALSE FALSE FALSE FALSE TRUE FALSE TRUE TRUE] -> w144
          frame "Low Bar", Default {
          }
          frame "Rough Terrain" {
          }
          frame "Moat" {
          }
          frame "Rock Wall" {
          }
          frame "Ramparts" {
          }
          frame "Cheval de Frise" {
          }
          frame "Portcullis" {
          }
          frame "Sally Port" {
          }
          frame "Drawbridge" {
          }
        }
        n80 = call-poly <userlib>:"Drive Loop Command.vi"("Distance"=140.0, "Absolute Angle? 4"=TRUE, "Angle 3"=w132, "Power 3"=w135, "Drive Loop Cluster"=w134) -> ()  [unwired: 7 in]
        n81 = Select(t=Auto_2_Control."Stop", s=w144, f=Auto_2_Control."Defense Crossing Detection") -> (s? t:f=w141:T4)
        n82 = shared-variable ".\\Shared.lvlib\\Encoder Distance"() -> (w140:dbl)  [unwired: 1 in, 1 out]
      }
      frame "Defense Crossing Detection" {
        # "or latch for hi/lo detection"
        # "Global Hi/Lo Peak\nand Portcullis Hold Values"
        # "Global Hi/Lo Peaks"
        # "Change State?"
        # "Encoder Count"
        # "Held Encoder Count"
        n83 = Unbundle By Name(w163) -> ("IMU Pitch"=w177:dbl, "Defense To Cross"=w176:T1, "Initial Position"=w175:T2, "IMU Roll"=w171:dbl)
        n84 = case shown="\"1\", Default" w175 {
          tunnel: [w195 w196 w197 w198 w199] -> w185
          frame "1", Default {
            n85 = shared-variable ".\\Auto QCP Variables.lvlib\\Position Offset_1"() -> (w195:dbl)  [unwired: 1 in, 1 out]
          }
          frame "2" {
            n86 = shared-variable ".\\Auto QCP Variables.lvlib\\Position Offset_2"() -> (w196:dbl)  [unwired: 1 in, 1 out]
          }
          frame "3" {
            n87 = shared-variable ".\\Auto QCP Variables.lvlib\\Position Offset_3"() -> (w197:dbl)  [unwired: 1 in, 1 out]
          }
          frame "4" {
            n88 = shared-variable ".\\Auto QCP Variables.lvlib\\Position Offset_4"() -> (w198:dbl)  [unwired: 1 in, 1 out]
          }
          frame "5" {
            n89 = shared-variable ".\\Auto QCP Variables.lvlib\\Position Offset_5"() -> (w199:dbl)  [unwired: 1 in, 1 out]
          }
        }
        n90 = feedback #1() -> (w167:T7)
        n91 = feedback #2() -> (w179:dbl)
        n92 = feedback #3() -> (w164:dbl)
        n93 = feedback #4() -> (w173:bool)
        "Pitch Up Detected" <- w173
        n94 = feedback #5() -> (w170:bool)
        "Pitch Down Detected" <- w170
        n95 = case shown="\"Rough Terrain\"" w176 {
          tunnel: w169 -> [w204 w208 w233 w262 w266 _ w307 _ _]
          tunnel: w191 -> [w202 w209 _ _ _ _ w303 _ _]
          tunnel: [w203 w207 w214 w241 w275 _ w305 _ FALSE] -> w189
          tunnel: [w202 w209 w231 w260 w292 _ w303 _ _] -> w190
          tunnel: [_ _ 0.0 0.0 w282 w298 0.0 ("Double") _ _] -> w184
          tunnel: w177 -> [_ _ w221 w251 w283 _ _ _ _]
          tunnel: w181 -> [_ _ _ _ _ _ _ _ _]
          tunnel: [_ _ w225 w254 w286 _ _ _ _] -> w180
          tunnel: w179 -> [_ _ w229 w258 w291 _ _ _ _]
          tunnel: [_ _ w224 w253 w287 _ w302 _ _] -> w178
          tunnel: w164 -> [_ _ w228 w257 w290 _ w306 _ _]
          tunnel: [_ _ w215 w245 w279 _ _ _ _] -> w174
          tunnel: w173 -> [_ _ w216 w246 w278 _ _ _ _]
          tunnel: [_ _ w212 w239 w277 _ _ _ _] -> w172
          tunnel: w170 -> [_ _ w211 w238 w276 _ _ _ _]
          tunnel: w171 -> [_ _ _ _ w272 _ _ _ _]
          tunnel: [w200 w205 _ _ _ _ _ _ _] -> w168
          tunnel: w167 -> [_ _ _ _ _ _ w310 _ _]
          tunnel: [_ _ _ _ _ _ w309 _ _] -> w166
          tunnel: w165 -> [_ _ _ _ _ _ w308 _ _]
          tunnel: w163 -> [_ _ _ _ _ _ w301 _ _]
          frame "Low Bar", Default {
            n96 = shared-variable ".\\Auto QCP Variables.lvlib\\Low Goal Enc"() -> (w201:dbl)  [unwired: 1 in, 1 out]
            n97 = Add(x=w201, y=w202) -> (x+y=w200:dbl)
            n98 = Greater Or Equal?(x=w204, y=w200) -> (x >= y?=w203:bool)
          }
          frame "Rough Terrain" {
            n99 = shared-variable ".\\Auto QCP Variables.lvlib\\Rough Terrain Enc"() -> (w206:dbl)  [unwired: 1 in, 1 out]
            n100 = Add(x=w206, y=w209) -> (x+y=w205:dbl)
            n101 = Greater Or Equal?(x=w208, y=w205) -> (x >= y?=w207:bool)
          }
          frame "Moat" {
            n102 = shared-variable ".\\Shared.lvlib\\IMU Pitch"() -> (w236:dbl)  [unwired: 1 in, 1 out]
            n103 = Subtract(x=w236, y=w221) -> (x-y=w237:dbl)
            n104 = Greater?(x=w237, y=w229) -> (0:w227:bool)
            n105 = Less?(x=w237, y=w228) -> (x < y?=w226:bool)
            n106 = shared-variable ".\\Auto QCP Variables.lvlib\\Moat Pitch"() -> (w223:dbl)  [unwired: 1 in, 1 out]
            n107 = Select(t=w237, s=w227, f=w229) -> (s? t:f=w225:dbl)
            n108 = Select(t=w237, s=w226, f=w228) -> (s? t:f=w224:dbl)
            n109 = Negate(x=w223) -> (-x=w222:dbl)
            n110 = shared-variable ".\\Auto QCP Variables.lvlib\\Moat Pitch T"() -> (w218:dbl)  [unwired: 1 in, 1 out]
            n111 = Greater?(x=w225, y=w223) -> (0:w220:bool)
            n112 = Less?(x=w224, y=w222) -> (x < y?=w219:bool)
            n113 = call <userlib>:"Stable.vi"("Eval Period (sec)"=w218, "Signal Input"=w220) -> ("Stable"=w217:bool)  [unwired: 9 in]
            n114 = call <userlib>:"Stable.vi"("Eval Period (sec)"=w218, "Signal Input"=w219) -> ("Stable"=w210:bool)  [unwired: 9 in]
            n115 = Or(x=w217, y=w216) -> (x .or. y?=w215:bool)
            n116 = Or(x=w211, y=w210) -> (x .or. y?=w212:bool)
            n117 = And(x=w215, y=w212) -> (x .and. y?=w213:bool)
            n118 = shared-variable ".\\Auto QCP Variables.lvlib\\Moat Enc"() -> (w235:dbl)  [unwired: 1 in, 1 out]
            n119 = call "Sample And Hold.vi"("Signal"=w233, "Condition"=w213) -> ("Signal Out"=w234:dbl)  [unwired: 9 in]
            n120 = Add(x=w234, y=w235) -> (x+y=w231:dbl)
            n121 = Greater Or Equal?(x=w233, y=w231) -> (x >= y?=w232:bool)
            n122 = And(x=w232, y=w213) -> (x .and. y?=w214:bool)
          }
          frame "Rock Wall" {
            n123 = shared-variable ".\\Shared.lvlib\\IMU Pitch"() -> (w264:dbl)  [unwired: 1 in, 1 out]
            n124 = Subtract(x=w264, y=w251) -> (x-y=w265:dbl)
            n125 = Greater?(x=w265, y=w258) -> (0:w256:bool)
            n126 = Less?(x=w265, y=w257) -> (x < y?=w255:bool)
            n127 = shared-variable ".\\Auto QCP Variables.lvlib\\Rockwall Pitch"() -> (w244:dbl)  [unwired: 1 in, 1 out]
            n128 = shared-variable ".\\Auto QCP Variables.lvlib\\Rockwall Pitch T"() -> (w248:dbl)  [unwired: 1 in, 1 out]
            n129 = Select(t=w265, s=w256, f=w258) -> (s? t:f=w254:dbl)
            n130 = Select(t=w265, s=w255, f=w257) -> (s? t:f=w253:dbl)
            n131 = Negate(x=w244) -> (-x=w252:dbl)
            n132 = Greater?(x=w254, y=w244) -> (0:w250:bool)
            n133 = Less?(x=w253, y=w252) -> (x < y?=w249:bool)
            n134 = call <userlib>:"Stable.vi"("Eval Period (sec)"=w248, "Signal Input"=w250) -> ("Stable"=w247:bool)  [unwired: 9 in]
            n135 = call <userlib>:"Stable.vi"("Eval Period (sec)"=w248, "Signal Input"=w249) -> ("Stable"=w242:bool)  [unwired: 9 in]
            n136 = Or(x=w247, y=w246) -> (x .or. y?=w245:bool)
            n137 = Or(x=w242, y=w238) -> (x .or. y?=w239:bool)
            n138 = shared-variable ".\\Auto QCP Variables.lvlib\\Rockwall Enc"() -> (w243:dbl)  [unwired: 1 in, 1 out]
            n139 = And(x=w245, y=w239) -> (x .and. y?=w240:bool)
            n140 = call "Sample And Hold.vi"("Signal"=w262, "Condition"=w240) -> ("Signal Out"=w263:dbl)  [unwired: 9 in]
            n141 = Add(x=w263, y=w243) -> (x+y=w260:dbl)
            n142 = Greater Or Equal?(x=w262, y=w260) -> (x >= y?=w261:bool)
            n143 = And(x=w261, y=w240) -> (x .and. y?=w241:bool)
          }
          frame "Ramparts" {
            n144 = shared-variable ".\\Shared.lvlib\\IMU Pitch"() -> (w297:dbl)  [unwired: 1 in, 1 out]
            n145 = shared-variable ".\\Shared.lvlib\\IMU Roll"() -> (w273:dbl)  [unwired: 1 in, 1 out]
            n146 = Subtract(x=w297, y=w283) -> (x-y=w270:dbl)
            n147 = Subtract(x=w273, y=w272) -> (x-y=w271:dbl)
            n148 = Subtract(x=w270, y=w271) -> (x-y=w269:dbl)
            n149 = shared-variable ".\\Auto QCP Variables.lvlib\\Ramparts Pitch"() -> (w284:dbl)  [unwired: 1 in, 1 out]
            n150 = Less?(x=w269, y=w290) -> (x < y?=w288:bool)
            n151 = Greater?(x=w269, y=w291) -> (0:w289:bool)
            n152 = shared-variable ".\\Auto QCP Variables.lvlib\\Ramparts Pitch T"() -> (w267:dbl)  [unwired: 1 in, 1 out]
            n153 = Select(t=w269, s=w288, f=w290) -> (s? t:f=w287:dbl)
            n154 = Select(t=w269, s=w289, f=w291) -> (s? t:f=w286:dbl)
            n155 = Negate(x=w284) -> (-x=w285:dbl)
            n156 = Less?(x=w287, y=w285) -> (x < y?=w281:bool)
            n157 = Greater?(x=w286, y=w284) -> (0:w296:bool)
            n158 = call <userlib>:"Stable.vi"("Eval Period (sec)"=w267, "Signal Input"=w281) -> ("Stable"=w280:bool)  [unwired: 9 in]
            n159 = call <userlib>:"Stable.vi"("Eval Period (sec)"=w267, "Signal Input"=w296) -> ("Stable"=w268:bool)  [unwired: 9 in]
            n160 = Or(x=w278, y=w280) -> (x .or. y?=w279:bool)
            n161 = Or(x=w268, y=w276) -> (x .or. y?=w277:bool)
            n162 = shared-variable ".\\Auto QCP Variables.lvlib\\Ramparts Enc"() -> (w295:dbl)  [unwired: 1 in, 1 out]
            n163 = And(x=w279, y=w277) -> (x .and. y?=w274:bool)
            n164 = call "Sample And Hold.vi"("Signal"=w266, "Condition"=w274) -> ("Signal Out"=w294:dbl)  [unwired: 9 in]
            n165 = shared-variable ".\\Auto QCP Variables.lvlib\\Ramparts Offset"() -> (w282:dbl)  [unwired: 1 in, 1 out]
            n166 = Add(x=w294, y=w295) -> (x+y=w292:dbl)
            n167 = Greater Or Equal?(x=w266, y=w292) -> (x >= y?=w293:bool)
            n168 = And(x=w274, y=w293) -> (x .and. y?=w275:bool)
          }
          frame "Cheval de Frise" {
            n169 = shared-variable ".\\Auto QCP Variables.lvlib\\See Saw Offset"() -> (w298:dbl)  [unwired: 1 in, 1 out]
          }
          frame "Portcullis" {
            n170 = Unbundle By Name(w301) -> ("Intake Command Cluster"=w299:T18, "Drive Loop Cluster"=w300:T15)
            n171 = case shown="\"Cross\"" w310 {
              selector: w310 -> [w324 _ w340 _ w356]
              tunnel: [w326 PortcullisStates."Pause" w342 PortcullisStates."Finish Cross" w356] -> w309
              tunnel: w300 -> [_ _ _ w343 _]
              tunnel: w308 -> [_ _ _ w346 _]
              tunnel: w307 -> [w316 _ _ _ w354]
              tunnel: w306 -> [w317 _ w333 _ _]
              tunnel: w303 -> [w322 _ _ _ w355]
              tunnel: [FALSE FALSE FALSE FALSE w352] -> w305
              tunnel: [w316 w330 w333 0.0 ("Double") 0.0 ("Double")] -> w302
              tunnel: w299 -> [_ w327 _ _ _]
              frame "Drive up to Portcullis", Default {
                n172 = Subtract(x=w316, y=w322) -> (x-y=w321:dbl)
                n173 = Greater Or Equal?(x=w321, y="Portcullis Point") -> (x >= y?=w319:bool)
                n174 = Subtract(x=w316, y=w317) -> (x-y=w315:dbl)
                n175 = call <userlib>:"Deadzone.vi"("Deadzone"="Encoder not moving val", "Input Signal"=w315) -> ("In Deadzone"=w314:bool)  [unwired: 1 out]
                n176 = call <userlib>:"Stable.vi"("Eval Period (sec)"="Eval Period for Port", "Signal Input"=w314) -> ("Stable"=w311:bool)  [unwired: 9 in]
                n177 = Or(x=w311, y=w319) -> (x .or. y?=w318:bool)
                n178 = Select(t=PortcullisStates."Intake Up", s=w318, f=w324) -> (s? t:f=w326:T7)
              }
              frame "Intake Up" {
                n179 = call-poly <userlib>:"Pneumatics Command Set.vi"("Solenoid Command"=Pneumatics_Command."Reverse", "Cluster"=w327) -> ()  [unwired: 9 in, 1 out]
                n180 = Get Date/Time In Seconds() -> (seconds since 1Jan1904=w331:timestamp)
                n181 = To Double Precision Float(number=w331) -> (double precision float=w330:dbl)
              }
              frame "Pause" {
                n182 = Get Date/Time In Seconds() -> (seconds since 1Jan1904=w338:timestamp)
                n183 = To Double Precision Float(number=w338) -> (double precision float=w337:dbl)
                n184 = Subtract(x=w337, y=w333) -> (x-y=w336:dbl)
                n185 = Greater Or Equal?(x=w336, y="Encoder Pause") -> (x >= y?=w334:bool)
                n186 = Select(t=PortcullisStates."Cross", s=w334, f=w340) -> (s? t:f=w342:T7)
              }
              frame "Cross" {
                n187 = call-poly <userlib>:"Drive Loop Command.vi"("Absolute Angle?"=TRUE, "Angle"=w346, "Power"="Portcullis Cross Power", "Drive Loop Cluster"=w343) -> ()  [unwired: 8 in]
              }
              frame "Finish Cross" {
                # "probs = to low bar"
                n188 = Add(x=w355, y="Dist cross") -> (x+y=w353:dbl)
                n189 = Greater Or Equal?(x=w354, y=w353) -> (x >= y?=w352:bool)
              }
            }
          }
          frame "Sally Port" {
          }
          frame "Drawbridge" {
          }
        }
        n190 = feedback-in #1(w166) -> ()
        n191 = feedback-in #2(w180) -> ()
        n192 = feedback-in #3(w178) -> ()
        n193 = feedback-in #4(w174) -> ()
        n194 = feedback-in #5(w172) -> ()
        n195 = Add(x=w184, y=w185) -> (x+y=w183:dbl)
        n196 = Select(t=Auto_2_Control."Drive Forward Past Defense", s=w189, f=w194) -> (s? t:f=w193:T4)
        n197 = Select(t=w169, s=w189, f=w190) -> (s? t:f=w188:dbl)
        n198 = Bundle By Name(cluster=cluster{"X":dbl, "Y":dbl} {"X"=0.0, "Y"=0.0} ("input cluster"), "X"=w183, "Y"=0.0) -> (w186:cluster{"X":dbl, "Y":dbl})
      }
      frame "Drive Forward Past Defense" {
        n199 = Unbundle By Name(w363) -> ("Y"=w371:dbl)
        n200 = shared-variable ".\\Shared.lvlib\\Encoder Distance"() -> (w374:dbl)  [unwired: 1 in, 1 out]
        n201 = shared-variable ".\\Auto QCP Variables.lvlib\\Courtyard Power"() -> (w358:dbl)  [unwired: 1 in, 1 out]
        n202 = Unbundle By Name(w367) -> ("Drive Loop Cluster"=w360:T15, "Goal Target"=w366:T3, "IMU Yaw"=w362:dbl, "Initial Position"=w365:T2)
        n203 = case shown="\"Left Goal\"" w366 {
          tunnel: w365 -> [w390 w404 _]
          tunnel: w377 -> [w389 w403 _]
          tunnel: [w388 w402 Auto_2_Control."Stop"] -> w376
          tunnel: Auto_2_Control."Turn to Rally Pt" ("t") -> [w387 w401 _]
          tunnel: w372 -> [w386 w400 _]
          tunnel: w374 -> [w382 w396 _]
          tunnel: [w385 w399 TRUE] -> w373
          tunnel: [w384 w398 0.0 ("Double")] -> w368
          tunnel: [w383 w397 _] -> w364
          frame "Left Goal" {
            n204 = case shown="\"1\", Default" w390 {
              tunnel: [w391 w392 w393 w394 0.0 ("Double")] -> w384
              frame "1", Default {
                n205 = shared-variable ".\\Auto QCP Variables.lvlib\\Drive Forward Pos_1l"() -> (w391:dbl)  [unwired: 1 in, 1 out]
              }
              frame "2" {
                n206 = shared-variable ".\\Auto QCP Variables.lvlib\\Drive Forward Pos_2l"() -> (w392:dbl)  [unwired: 1 in, 1 out]
              }
              frame "3" {
                n207 = shared-variable ".\\Auto QCP Variables.lvlib\\Drive Forward Pos_3l"() -> (w393:dbl)  [unwired: 1 in, 1 out]
              }
              frame "4" {
                n208 = shared-variable ".\\Auto QCP Variables.lvlib\\Drive Forward Pos_4l"() -> (w394:dbl)  [unwired: 1 in, 1 out]
              }
              frame "5" {
              }
            }
            n209 = Add(x=w384, y=w386) -> (x+y=w383:dbl)
            n210 = Greater Or Equal?(x=w382, y=w383) -> (x >= y?=w385:bool)
            n211 = Select(t=w387, s=w385, f=w389) -> (s? t:f=w388:T4)
          }
          frame "Right Goal" {
            n212 = case shown="\"2\"" w404 {
              tunnel: [0.0 ("Double") w406 w407 w408 w409] -> w398
              frame "1", Default {
              }
              frame "2" {
                n213 = shared-variable ".\\Auto QCP Variables.lvlib\\Drive Forward Pos_2r"() -> (w406:dbl)  [unwired: 1 in, 1 out]
              }
              frame "3" {
                n214 = shared-variable ".\\Auto QCP Variables.lvlib\\Drive Forward Pos_3r"() -> (w407:dbl)  [unwired: 1 in, 1 out]
              }
              frame "4" {
                n215 = shared-variable ".\\Auto QCP Variables.lvlib\\Drive Forward Pos_4r"() -> (w408:dbl)  [unwired: 1 in, 1 out]
              }
              frame "5" {
                n216 = shared-variable ".\\Auto QCP Variables.lvlib\\Drive Forward Pos_5r"() -> (w409:dbl)  [unwired: 1 in, 1 out]
              }
            }
            n217 = Add(x=w398, y=w400) -> (x+y=w397:dbl)
            n218 = Greater Or Equal?(x=w396, y=w397) -> (x >= y?=w399:bool)
            n219 = Select(t=w401, s=w399, f=w403) -> (s? t:f=w402:T4)
          }
          frame "Stop", Default {
          }
        }
        n220 = call-poly <userlib>:"Drive Loop Command.vi"("Distance"=140.0, "Absolute Angle? 4"=TRUE ("Absolute Angle?"), "Angle 3"=w362, "Power 3"=w358, "Drive Loop Cluster"=w360) -> ()  [unwired: 7 in]
        n221 = case shown="True" w373 {
          tunnel: [w378 w380] -> w369
          tunnel: w371 -> [w378 w381]
          tunnel: w368 -> [_ w379]
          frame False {
          }
          frame True {
            n222 = Add(x=w379, y=w381) -> (x+y=w380:dbl)
          }
        }
        n223 = Bundle By Name(cluster=w363, "Y"=w369) -> (w370:cluster{"X":dbl, "Y":dbl})
      }
      frame "Turn to Rally Pt" {
        n224 = Unbundle By Name(w431) -> ("Intake Command Cluster"=w413:T18, "Drive Loop Cluster"=w430:T15, "Goal Target"=w429:T3, "IMU Yaw"=w417:dbl, "Initial Position"=w428:T2)
        n225 = case shown="\"Right Goal\"" w429 {
          tunnel: w428 -> [w443 w459]
          tunnel: w417 -> [_ _]
          tunnel: w432 -> [w442 w458]
          tunnel: [w442 w458] -> w422
          tunnel: [w441 w457] -> w421
          frame "Left Goal", Default {
            n226 = case shown="\"2\"" w443 {
              tunnel: [w444 w447 w450 w453 cluster{"Double":dbl, "Double":dbl} {"Double"=0.0, "Double"=0.0}] -> w441
              frame "1" {
                n227 = shared-variable ".\\Auto QCP Variables.lvlib\\Rally Pt 1 X"() -> (w446:dbl)  [unwired: 1 in, 1 out]
                n228 = shared-variable ".\\Auto QCP Variables.lvlib\\Rally Pt 1 Y"() -> (w445:dbl)  [unwired: 1 in, 1 out]
                n229 = Bundle("Double"=w446, "Double"=w445) -> (w444:cluster{"Double":dbl, "Double":dbl})  [unwired: 1 in]
              }
              frame "2" {
                n230 = shared-variable ".\\Auto QCP Variables.lvlib\\Rally Pt 2 X L"() -> (w449:dbl)  [unwired: 1 in, 1 out]
                n231 = shared-variable ".\\Auto QCP Variables.lvlib\\Rally Pt 2 Y L"() -> (w448:dbl)  [unwired: 1 in, 1 out]
                n232 = Bundle("Double"=w449, "Double"=w448) -> (w447:cluster{"Double":dbl, "Double":dbl})  [unwired: 1 in]
              }
              frame "3", Default {
                n233 = shared-variable ".\\Auto QCP Variables.lvlib\\Rally Pt 3 X L"() -> (w452:dbl)  [unwired: 1 in, 1 out]
                n234 = shared-variable ".\\Auto QCP Variables.lvlib\\Rally Pt 3 Y L"() -> (w451:dbl)  [unwired: 1 in, 1 out]
                n235 = Bundle("Double"=w452, "Double"=w451) -> (w450:cluster{"Double":dbl, "Double":dbl})  [unwired: 1 in]
              }
              frame "4" {
                n236 = shared-variable ".\\Auto QCP Variables.lvlib\\Rally Pt 4 X L"() -> (w455:dbl)  [unwired: 1 in, 1 out]
                n237 = shared-variable ".\\Auto QCP Variables.lvlib\\Rally Pt 4 Y L"() -> (w454:dbl)  [unwired: 1 in, 1 out]
                n238 = Bundle("Double"=w455, "Double"=w454) -> (w453:cluster{"Double":dbl, "Double":dbl})  [unwired: 1 in]
              }
              frame "5" {
              }
            }
          }
          frame "Right Goal" {
            n239 = case shown="\"5\"" w459 {
              tunnel: [w461 w462 w465 w468 w471] -> w457
              frame "1" {
                w460 = 0.0 ("Rally Pt 2 X L")
                n240 = Bundle("Rally Pt 2 X L"=w460, "Rally Pt 2 X L"=w460) -> (w461:T24)  [unwired: 1 in]
              }
              frame "2" {
                n241 = shared-variable ".\\Auto QCP Variables.lvlib\\Rally Pt 2 X R"() -> (w464:dbl)  [unwired: 1 in, 1 out]
                n242 = shared-variable ".\\Auto QCP Variables.lvlib\\Rally Pt 2 Y R"() -> (w463:dbl)  [unwired: 1 in, 1 out]
                n243 = Bundle("Double"=w464, "Double"=w463) -> (w462:cluster{"Double":dbl, "Double":dbl})  [unwired: 1 in]
              }
              frame "3", Default {
                n244 = shared-variable ".\\Auto QCP Variables.lvlib\\Rally Pt 3 X R"() -> (w467:dbl)  [unwired: 1 in, 1 out]
                n245 = shared-variable ".\\Auto QCP Variables.lvlib\\Rally Pt 3 Y R"() -> (w466:dbl)  [unwired: 1 in, 1 out]
                n246 = Bundle("Double"=w467, "Double"=w466) -> (w465:cluster{"Double":dbl, "Double":dbl})  [unwired: 1 in]
              }
              frame "4" {
                n247 = shared-variable ".\\Auto QCP Variables.lvlib\\Rally Pt 4 X R"() -> (w470:dbl)  [unwired: 1 in, 1 out]
                n248 = shared-variable ".\\Auto QCP Variables.lvlib\\Rally Pt 4 Y R"() -> (w469:dbl)  [unwired: 1 in, 1 out]
                n249 = Bundle("Double"=w470, "Double"=w469) -> (w468:cluster{"Double":dbl, "Double":dbl})  [unwired: 1 in]
              }
              frame "5" {
                n250 = shared-variable ".\\Auto QCP Variables.lvlib\\Rally Pt 5 X"() -> (w473:dbl)  [unwired: 1 in, 1 out]
                n251 = shared-variable ".\\Auto QCP Variables.lvlib\\Rally Pt 5 Y"() -> (w472:dbl)  [unwired: 1 in, 1 out]
                n252 = Bundle("Double"=w473, "Double"=w472) -> (w471:cluster{"Double":dbl, "Double":dbl})  [unwired: 1 in]
              }
            }
          }
        }
        n253 = call-poly <userlib>:"Pneumatics Command Set.vi"("Solenoid Command"=Pneumatics_Command."Forward", "Cluster"=w413) -> ()  [unwired: 9 in, 1 out]
        n254 = call "Distance and Angle.vi"("END"=w421, "START"=w422) -> ("Angle"=w415:dbl, "Distance"=w420:dbl)  [unwired: 8 in]
        n255 = shared-variable ".\\Shared.lvlib\\IMU Yaw"() -> (w416:dbl)  [unwired: 1 in, 1 out]
        n256 = Subtract(x=w416, y=w417) -> (x-y=w423:dbl)
        n257 = call "Wrapped To Absolute.vi"("Desired Angle"=w415, "Wrapped Value"=w423) -> ("Output"=w419:dbl)  [unwired: 8 in, 1 out]
        n258 = Add(x=w419, y=w417) -> (x+y=w418:dbl)
        n259 = Subtract(x=w418, y=w416) -> (x-y=w425:dbl)
        n260 = Absolute Value(x=w425) -> (abs(x)=w424:dbl)
        n261 = Less Or Equal?(x=w424, y=5.0) -> (x <= y?=w426:bool)
        n262 = case shown="True" w426 {
          tunnel: [Auto_2_Control."Drive to Rally Pt" ("t") Auto_2_Control."Complete Rally Pt Turn" ("t")] -> w434
          tunnel: w430 -> [_ w436]
          tunnel: w418 -> [_ w439]
          frame False {
          }
          frame True {
            n263 = call-poly <userlib>:"Drive Loop Command.vi"("Absolute Angle? in"=TRUE, "Angle in"=w439, "Power in"=0.7, "Drive Loop Cluster"=w436) -> ()  [unwired: 8 in]
          }
        }
        n264 = shared-variable ".\\Shared.lvlib\\Rally Point Distance"(w420) -> ()  [unwired: 1 in, 1 out]
        n265 = shared-variable ".\\Shared.lvlib\\Encoder Distance"() -> (w433:dbl)  [unwired: 1 in, 1 out]
      }
      frame "Complete Rally Pt Turn" {
        n266 = shared-variable ".\\Shared.lvlib\\IMU Yaw"() -> (w486:dbl)  [unwired: 1 in, 1 out]
        n267 = Subtract(x=w486, y=w474) -> (x-y=w485:dbl)
        n268 = shared-variable ".\\Auto QCP Variables.lvlib\\Turn to Rally Pt Tol"() -> (w476:dbl)  [unwired: 1 in, 1 out]
        n269 = Absolute Value(x=w485) -> (abs(x)=w484:dbl)
        n270 = shared-variable ".\\Auto QCP Variables.lvlib\\Turn to Rally Pt Eval"() -> (w475:dbl)  [unwired: 1 in, 1 out]
        n271 = Less Or Equal?(x=w484, y=w476) -> (x <= y?=w483:bool)
        n272 = call <userlib>:"Stable.vi"("Eval Period (sec)"=w475, "Signal Input"=w483) -> ("Stable"=w480:bool)  [unwired: 9 in]
        n273 = Select(t=Auto_2_Control."Drive to Rally Pt", s=w480, f=w479) -> (s? t:f=w482:T4)
        n274 = shared-variable ".\\Shared.lvlib\\Encoder Distance"() -> (w478:dbl)  [unwired: 1 in, 1 out]
      }
      frame "Drive to Rally Pt" {
        n275 = Unbundle By Name(w492) -> ("Drive Loop Cluster"=w487:T15)
        n276 = shared-variable ".\\Shared.lvlib\\Rally Point Distance"() -> (w493:dbl)  [unwired: 1 in, 1 out]
        n277 = Add(x=w493, y=w495) -> (x+y=w491:dbl)
        n278 = call-poly <userlib>:"Drive Loop Command.vi"("Absolute Angle?"=TRUE, "Angle"=w488, "Power"=0.7, "Drive Loop Cluster"=w487) -> ()  [unwired: 8 in]
      }
      frame "Finish Drive to Rally Pt" {
        n279 = shared-variable ".\\Shared.lvlib\\Encoder Distance"() -> (w499:dbl)  [unwired: 1 in, 1 out]
        n280 = Greater Or Equal?(x=w499, y=w498) -> (x >= y?=w501:bool)
        n281 = Select(t=Auto_2_Control."Turn to Tower", s=w501, f=w502) -> (s? t:f=w504:T4)
      }
      frame "Turn to Tower" {
        # "What is this for?"
        n282 = Unbundle By Name(w519) -> ("Drive Loop Cluster"=w505:T15, "Goal Target"=w518:T3, "IMU Yaw"=w514:dbl)
        n283 = case shown="\"Left Goal\", Default" w518 {
          tunnel: [w524 w526] -> w517
          tunnel: [w523 w525] -> w516
          frame "Left Goal", Default {
            n284 = shared-variable ".\\Auto QCP Variables.lvlib\\Tower Loc L X"() -> (w524:dbl)  [unwired: 1 in, 1 out]
            n285 = shared-variable ".\\Auto QCP Variables.lvlib\\Tower Loc L Y"() -> (w523:dbl)  [unwired: 1 in, 1 out]
          }
          frame "Right Goal" {
            n286 = shared-variable ".\\Auto QCP Variables.lvlib\\Tower Loc R X"() -> (w526:dbl)  [unwired: 1 in, 1 out]
            n287 = shared-variable ".\\Auto QCP Variables.lvlib\\Tower Loc R Y"() -> (w525:dbl)  [unwired: 1 in, 1 out]
          }
        }
        n288 = shared-variable ".\\Shared.lvlib\\IMU Yaw"() -> (w515:dbl)  [unwired: 1 in, 1 out]
        n289 = Bundle("Double"=w517, "Double"=w516) -> (w509:cluster{"Double":dbl, "Double":dbl})  [unwired: 1 in]
        n290 = Subtract(x=w515, y=w514) -> (x-y=w512:dbl)
        n291 = call "Distance and Angle.vi"("END"=w509, "START"=w510) -> ("Angle"=w513:dbl, "Distance"=w520:dbl)  [unwired: 8 in]
        n292 = call "Wrapped To Absolute.vi"("Desired Angle"=w513, "Wrapped Value"=w512) -> ("Output"=w511:dbl)  [unwired: 8 in, 1 out]
        n293 = Add(x=w514, y=w511) -> (x+y=w508:dbl)
        n294 = shared-variable ".\\Shared.lvlib\\Tower Distance to Travel"(w520) -> ()  [unwired: 1 in, 1 out]
        n295 = call-poly <userlib>:"Drive Loop Command.vi"("Absolute Angle? in"=TRUE, "Angle in"=w508, "Power in"=1.0, "Drive Loop Cluster"=w505) -> ()  [unwired: 8 in]
        n296 = shared-variable ".\\Shared.lvlib\\Encoder Distance"() -> (w521:dbl)  [unwired: 1 in, 1 out]
      }
      frame "Complete Turn to Tower" {
        n297 = shared-variable ".\\Shared.lvlib\\IMU Yaw"() -> (w541:dbl)  [unwired: 1 in, 1 out]
        n298 = Subtract(x=w541, y=w536) -> (x-y=w540:dbl)
        n299 = shared-variable ".\\Auto QCP Variables.lvlib\\Turn to Tower Tol"() -> (w529:dbl)  [unwired: 1 in, 1 out]
        n300 = Absolute Value(x=w540) -> (abs(x)=w539:dbl)
        n301 = shared-variable ".\\Auto QCP Variables.lvlib\\Turn to Tower Eval"() -> (w528:dbl)  [unwired: 1 in, 1 out]
        n302 = shared-variable ".\\Auto QCP Variables.lvlib\\Camera Angle Good"() -> (w527:bool)  [unwired: 1 in, 1 out]
        n303 = Less Or Equal?(x=w539, y=w529) -> (x <= y?=w538:bool)
        n304 = call <userlib>:"Stable.vi"("Eval Period (sec)"=w528, "Signal Input"=w538) -> ("Stable"=w532:bool)  [unwired: 9 in]
        n305 = Or(x=w527, y=w532) -> (x .or. y?=w531:bool)
        n306 = Select(t=Auto_2_Control."Drive to Tower", s=w531, f=w535) -> (s? t:f=w534:T4)
        n307 = shared-variable ".\\Shared.lvlib\\Encoder Distance"() -> (w533:dbl)  [unwired: 1 in, 1 out]
      }
      frame "Drive to Tower" {
        # "Need for Max Tower Distance to Travel Removed and\nUNNECESSARY"
        n308 = Unbundle By Name(w544) -> ("Drive Loop Cluster"=w543:T15)
        n309 = call-poly <userlib>:"Drive Loop Command.vi"("Power 5"=1.0 ("Power 6"), "Drive Loop Cluster"=w543) -> ()  [unwired: 10 in]
        n310 = shared-variable ".\\Shared.lvlib\\Tower Distance to Travel"() -> (w545:dbl)  [unwired: 1 in, 1 out]
        n311 = shared-variable ".\\Shared.lvlib\\Encoder Distance"() -> (w549:dbl)  [unwired: 1 in, 1 out]
        n312 = Add(x=w545, y=w549) -> (x+y=w548:dbl)
      }
      frame "Complete Drive to Tower" {
        n313 = Unbundle By Name(w552) -> ("Goal Target"=w554:T3, "IMU Pitch"=w561:dbl)
        n314 = shared-variable ".\\Vision Variables.lvlib\\Valid"() -> (w551:bool)  [unwired: 1 in, 1 out]
        n315 = case shown="True" w551 {
          tunnel: w552 -> [_ w578]
          frame False {
          }
          frame True {
            n316 = Unbundle By Name(w578) -> ("Drive Loop Cluster"=w577:T15)
            n317 = call-poly <userlib>:"Drive Loop Command.vi"("Power 6"=1.0, "Drive Loop Cluster"=w577) -> ()  [unwired: 10 in]
          }
        }
        n318 = shared-variable ".\\Shared.lvlib\\IMU Pitch"() -> (w572:dbl)  [unwired: 1 in, 1 out]
        n319 = shared-variable ".\\Auto QCP Variables.lvlib\\Batter Pitch Thresh"() -> (w563:dbl)  [unwired: 1 in, 1 out]
        n320 = shared-variable ".\\Shared.lvlib\\Encoder Distance"() -> (w556:dbl)  [unwired: 1 in, 1 out]
        n321 = Subtract(x=w572, y=w561) -> (x-y=w559:dbl)
        n322 = case shown="\"Right Goal\"" w554 {
          tunnel: [w579 w580] -> w558
          frame "Left Goal", Default {
            n323 = shared-variable ".\\Auto QCP Variables.lvlib\\Tower Min Enc L"() -> (w579:dbl)  [unwired: 1 in, 1 out]
          }
          frame "Right Goal" {
            n324 = shared-variable ".\\Auto QCP Variables.lvlib\\Tower Min Enc R"() -> (w580:dbl)  [unwired: 1 in, 1 out]
          }
        }
        n325 = Greater?(x=w559, y=w563) -> (0:w571:bool)
        "Over Pitch Th" <- w571
        n326 = Greater Or Equal?(x=w556, y=w566) -> (x >= y?=w570:bool)
        n327 = Add(x=w557, y=w558) -> (x+y=w555:dbl)
        n328 = Greater Or Equal?(x=w556, y=w555) -> (x >= y?=w568:bool)
        "Over Encoder Distance" <- w568
        n329 = shared-variable ".\\Auto QCP Variables.lvlib\\Batter Pitch T"() -> (w562:dbl)  [unwired: 1 in, 1 out]
        n330 = And(x=w568, y=w571) -> (x .and. y?=w569:bool)
        n331 = call <userlib>:"Stable.vi"("Eval Period (sec)"=w562, "Signal Input"=w569) -> ("Stable"=w567:bool)  [unwired: 9 in]
        "Stable Over Pitch" <- w567
        n332 = Compound Arithmetic op=OR(w567, w570, "Override Pitch Detection") -> (w565:bool)
        n333 = Select(t=Auto_2_Control."Score", s=w565, f=w574) -> (s? t:f=w573:T4)
      }
      frame "Score" {
        n334 = Unbundle By Name(w586) -> ("intakeMotor"=w585:T8, "Drive Loop Cluster"=w584:T15, "Leave Tower?"=w583:bool)
        n335 = Get Date/Time In Seconds() -> (seconds since 1Jan1904=w598:timestamp)
        n336 = shared-variable ".\\Shared.lvlib\\IMU Yaw"() -> (w592:dbl)  [unwired: 1 in, 1 out]
        n337 = To Double Precision Float(number=w598) -> (double precision float=w597:dbl)
        n338 = call <vilib>:"WPI_MotorControlSetOutput.vi"("Output"=1.0, "MotorControlDevRef"=w585) -> ()  [unwired: 7 in, 3 out]
        n339 = Subtract(x=w597, y=w582) -> (x-y=w596:dbl)
        n340 = case shown="True" w581 {
          tunnel: w592 -> [_ w603]
          tunnel: w584 -> [_ w604]
          frame False {
          }
          frame True {
            # "This previously used an\nabused hold position+12\"\n\nIt now uses drive distance\nWith same settings except\nfor PID."
            n341 = call-poly <userlib>:"Drive Loop Command.vi"("Distance"=12.0, "Absolute Angle? 4"=TRUE, "Angle 3"=w603, "Power 3"=1.0 ("Power 4"), "Drive Loop Cluster"=w604) -> ()  [unwired: 7 in]
          }
        }
        n342 = Select(t=Auto_2_Control."Parallel to Position", s=w583, f=Auto_2_Control."Stop") -> (s? t:f=w589:T4)
        n343 = Greater Or Equal?(x=w596, y="Score Intake timer") -> (x >= y?=w595:bool)
        n344 = Select(t=w589, s=w595, f=w600) -> (s? t:f=w599:T4)
        n345 = shared-variable ".\\Shared.lvlib\\Encoder Distance"() -> (w591:dbl)  [unwired: 1 in, 1 out]
      }
      frame "Parallel to Position" {
        n346 = Unbundle By Name(w614) -> ("Drive Loop Cluster"=w606:T15, "intakeMotor"=w610:T8)
        n347 = call <vilib>:"WPI_MotorControlSetOutput.vi"("Output"=0.0, "MotorControlDevRef"=w610) -> ()  [unwired: 7 in, 3 out]
        n348 = call-poly <userlib>:"Drive Loop Command.vi"("Angle"=w608, "Power"="Backup Power", "Drive Loop Cluster"=w606) -> ()  [unwired: 9 in]
      }
      frame "Finish Backing Parallel to Pos" {
        n349 = Unbundle By Name(w640) -> ("IMU Yaw"=w620:dbl, "Return Position"=w639:T2, "Intake Command Cluster"=w615:T18)
        n350 = case shown="\"1\", Default" w639 {
          tunnel: [w648 w649 w650 w651 w652] -> w619
          frame "1", Default {
            n351 = shared-variable ".\\Auto QCP Variables.lvlib\\Position Offset_1"() -> (w648:dbl)  [unwired: 1 in, 1 out]
          }
          frame "2" {
            n352 = shared-variable ".\\Auto QCP Variables.lvlib\\Position Offset_2"() -> (w649:dbl)  [unwired: 1 in, 1 out]
          }
          frame "3" {
            n353 = shared-variable ".\\Auto QCP Variables.lvlib\\Position Offset_3"() -> (w650:dbl)  [unwired: 1 in, 1 out]
          }
          frame "4" {
            n354 = shared-variable ".\\Auto QCP Variables.lvlib\\Position Offset_4"() -> (w651:dbl)  [unwired: 1 in, 1 out]
          }
          frame "5" {
            n355 = shared-variable ".\\Auto QCP Variables.lvlib\\Position Offset_5"() -> (w652:dbl)  [unwired: 1 in, 1 out]
          }
        }
        n356 = Subtract(x=w622, y=w620) -> (x-y=w621:dbl)
        n357 = expression code="(x/180.0)*pi" "degrees to radians"(w621) -> (w623:dbl)
        n358 = Add(x=w630, y="Tower Backup Offset") -> (x+y=w643:dbl)
        n359 = Subtract(x=w643, y=w644) -> (x-y=w636:dbl)
        n360 = Sine & Cosine(0:w623) -> (1:w642:dbl, 2:w637:dbl)
        n361 = Multiply(x=w636, y=w642) -> (x*y=w641:dbl)
        "X pos" <- w641
        n362 = Multiply(x=w636, y=w637) -> (x*y=w635:dbl)
        n363 = Unbundle By Name(w632) -> ("X"=w624:dbl, "Y"=w625:dbl)
        "Y" <- w625
        n364 = Subtract(x=179.5 ("Defense to Wall"), y=w635) -> (x-y=w629:dbl)
        n365 = Subtract(x=w624, y=w619) -> (x-y=w638:dbl)
        "Desired X pos" <- w638
        n366 = Subtract(x=w629, y="Dist from Def") -> (x-y=w618:dbl)
        n367 = Greater Or Equal?(x=w641, y=w638) -> (x >= y?=w616:bool)
        n368 = Select(t=Auto_2_Control."Turn to Defense ", s=w616, f=w627) -> (s? t:f=w634:T4)
        n369 = Select(t=w618, s=w616, f=w625) -> (s? t:f=w628:dbl)
        n370 = case shown="True" w616 {
          tunnel: w615 -> [_ w646]
          frame False {
          }
          frame True {
            n371 = call-poly <userlib>:"Pneumatics Command Set.vi"("Solenoid Command"=Pneumatics_Command."Reverse", "Cluster"=w646) -> ()  [unwired: 9 in, 1 out]
          }
        }
        n372 = Bundle By Name(cluster=w632, "Y"=w628) -> (w631:cluster{"X":dbl, "Y":dbl})
      }
      frame "Turn to Defense " {
        n373 = Unbundle By Name(w666) -> ("IMU Yaw"=w659:dbl, "Drive Loop Cluster"=w653:T15, "Goal Target"=w663:T3)
        n374 = Equal?(x=w663, y=Goal_Selection."Left Goal") -> (x = y?=w664:bool)
        n375 = Select(t=180.0, s=w664, f=-180.0) -> (s? t:f=w665:dbl)
        n376 = Add(x=w665, y=w659) -> (x+y=w656:dbl)
        n377 = call-poly <userlib>:"Drive Loop Command.vi"("Absolute Angle? in"=TRUE, "Angle in"=w656, "Power in"=1.0, "Drive Loop Cluster"=w653) -> ()  [unwired: 8 in]
      }
      frame "Finish Turn to Def" {
        n378 = Unbundle By Name(w681) -> ("IMU Yaw"=w680:dbl)
        n379 = Subtract(x=w682, y=w680) -> (x-y=w679:dbl)
        n380 = Subtract(x=w679, y=w669) -> (x-y=w678:dbl)
        n381 = Absolute Value(x=w678) -> (abs(x)=w677:dbl)
        n382 = Less Or Equal?(x=w677, y=2.0 ("Finish Turn to Def Tol")) -> (x <= y?=w675:bool)
        n383 = call <userlib>:"Stable.vi"("Eval Period (sec)"=0.5 ("Finish Turn to Def Stable"), "Signal Input"=w675) -> ("Stable"=w673:bool)  [unwired: 9 in]
        n384 = disable-structure shown="Enabled" {
          disable-tunnel: [Auto_2_Control."Back to Defense" Auto_2_Control."Stop"] -> w671
          frame Disabled {
          }
          frame Enabled {
          }
        }
        n385 = Select(t=w671, s=w673, f=w670) -> (s? t:f=w672:T4)
        n386 = shared-variable ".\\Shared.lvlib\\Encoder Distance"() -> (w668:dbl)  [unwired: 1 in, 1 out]
      }
      frame "Back to Defense" {
        n387 = Unbundle By Name(w695) -> ("Drive Loop Cluster"=w686:T15, "Return Point"=w694:cluster{"X":dbl, "Y":dbl})
        n388 = Unbundle By Name(w693) -> ("Y"=w691:dbl)
        n389 = Add(x=w691, y=w692) -> (x+y=w690:dbl)
        n390 = shared-variable ".\\Auto QCP Variables.lvlib\\Courtyard Power"() -> (w689:dbl)  [unwired: 1 in, 1 out]
        n391 = call-poly <userlib>:"Drive Loop Command.vi"("Absolute Angle?"=TRUE, "Angle"=w688, "Power"=w689, "Drive Loop Cluster"=w686) -> ()  [unwired: 8 in]
      }
      frame "Finish Back to Defense" {
        n392 = Less Or Equal?(x=w699, y=w698) -> (x <= y?=w697:bool)
        n393 = Select(t=Auto_2_Control."Stop", s=w697, f=w703) -> (s? t:f=w701:T4)
      }
      frame "Stop" {
        n394 = Unbundle By Name(w709) -> ("Drive Loop Cluster"=w708:T15, "intakeMotor"=w705:T8)  [unwired: 2 out]
        n395 = call <vilib>:"WPI_MotorControlSetOutput.vi"("Output"=1.0, "MotorControlDevRef"=w705) -> ()  [unwired: 7 in, 3 out]
        n396 = case shown="True" w707 {
          tunnel: w708 -> [_ w714]
          frame False {
          }
          frame True {
            n397 = call-poly <userlib>:"Drive Loop Command.vi"("Power 4"=1.0, "Drive Loop Cluster"=w714) -> ()  [unwired: 10 in]
          }
        }
      }
    }
    "Current State" <- w92
    "Target Distance" <- w88
    "Desired Angle" <- w87
    "Robot Pitch" <- w82
    "XY Current" <- w95
    n398 = shared-variable ".\\Vision Variables.lvlib\\Valid"() -> (w81:bool)  [unwired: 1 in, 1 out]
    n399 = feedback #6() -> (w79:bool)
    "Camera Valid" <- w79
    n400 = Or(x=w79, y=w81) -> (x .or. y?=w80:bool)
    n401 = feedback-in #6(w80) -> ()
    n402 = node-c288() -> ()  [unwired: 1 in, 1 out]
  }
  n403 = node-c288(w46) -> ()  [unwired: 1 out]
